vi "Autonomous Independent.vi"() -> ()   [LabVIEW 2015]
doc: "This VI is called when autonomous begins, and will automatically be terminated when autonomous ends. You can carry out timed or sensor driven robot movement independently without needing to return to the caller."
uses:
  AutoStatesTypeDef.ctl
  Auton Defenses Enum.ctl
  <vilib>/Rock Robotics/WPI/Utilities/WPI_GetSetVariantRefNum.vi
  <vilib>/Rock Robotics/Network Tables/NT Read String.vi
  <vilib>/Rock Robotics/Network Tables/NT Write Numeric Array.vi
  <vilib>/Rock Robotics/Network Tables/NT Read Number.vi
  <vilib>/Rock Robotics/Network Tables/NT Write Number.vi
  Robot Values.vi
  Robot Global.vi
  <vilib>/Rock Robotics/Network Tables/NT Read Boolean.vi
  <vilib>/Rock Robotics/WPI/RobotDrive/WPI_RobotDriveArcadeDrive_Standard(NoSaturation).vi
panel:
  in  "PID gains 7":T1={"proportional gain (Kc)"=0.015, "integral time (Ti, min)"=0.0, "derivative time (Td, min)"=0.0}
  in  "PID gains 5":T1={"proportional gain (Kc)"=0.015, "integral time (Ti, min)"=0.0, "derivative time (Td, min)"=0.0}
  in  "PID gains 4":T1={"proportional gain (Kc)"=0.015, "integral time (Ti, min)"=0.0, "derivative time (Td, min)"=0.0}
  in  "PID gains 3":T1={"proportional gain (Kc)"=0.015, "integral time (Ti, min)"=0.0, "derivative time (Td, min)"=0.0}
  in  "Pos 5 Turn":dbl=180.0 format="%#_13g"
  in  "Pos 4 Turn":dbl=180.0 format="%#_13g"
  in  "Pos 3 Turn":dbl=180.0 format="%#_13g"
  in  "Pos 2 Turn":dbl=180.0 format="%#_13g"
  in  "Pos 5 Align":dbl=105.0 format="%#_13g"
  in  "Pos 4 Align":dbl=170.0 format="%#_13g"
  in  "Pos 3 Align":dbl=255.0 format="%#_13g"
  in  "Pos 2 Align":dbl=260.0 format="%#_13g"
  in  "Pos 5 Drive":dbl=-450.0 format="%#_13g"
  in  "Pos 4 Drive":dbl=-50.0 format="%#_13g"
  in  "Pos 3 Drive":dbl=-100.0 format="%#_13g"
  in  "Pos 2 Drive":dbl=-680.0 format="%#_13g"
  in  "PID gains 2":T1={"proportional gain (Kc)"=0.015, "integral time (Ti, min)"=0.0, "derivative time (Td, min)"=0.0}
  in  "Initial State":T2
  in  "Auton":T3={"Position"=enum."First", "Defense"=enum."Low Bar"}
  out "Current Movement, for debugging":T4 {"Y Joystick Value" scale=1.0..-1.0; "X Joystick Value" scale=-1.0..1.0}
  in  "Array of robot movements":T5(array[cluster])=[{"X Joystick Value"=0.39393939393939403, "Y Joystick Value"=0.0, "Delay (sec)"=1.0, "Movement Name"="turn"}, {"X Joystick Value"=-0.3737373737373737, "Y Joystick Value"=0.0, "Delay (sec)"=1.0, "Movement Name"="turn back"}] {"Y Joystick Value" scale=1.0..-1.0; "X Joystick Value" scale=-1.0..1.0}
  # "Be sure to right-click and choose Data Operations>>Make Current Value default if you want to save the array values with the VI"
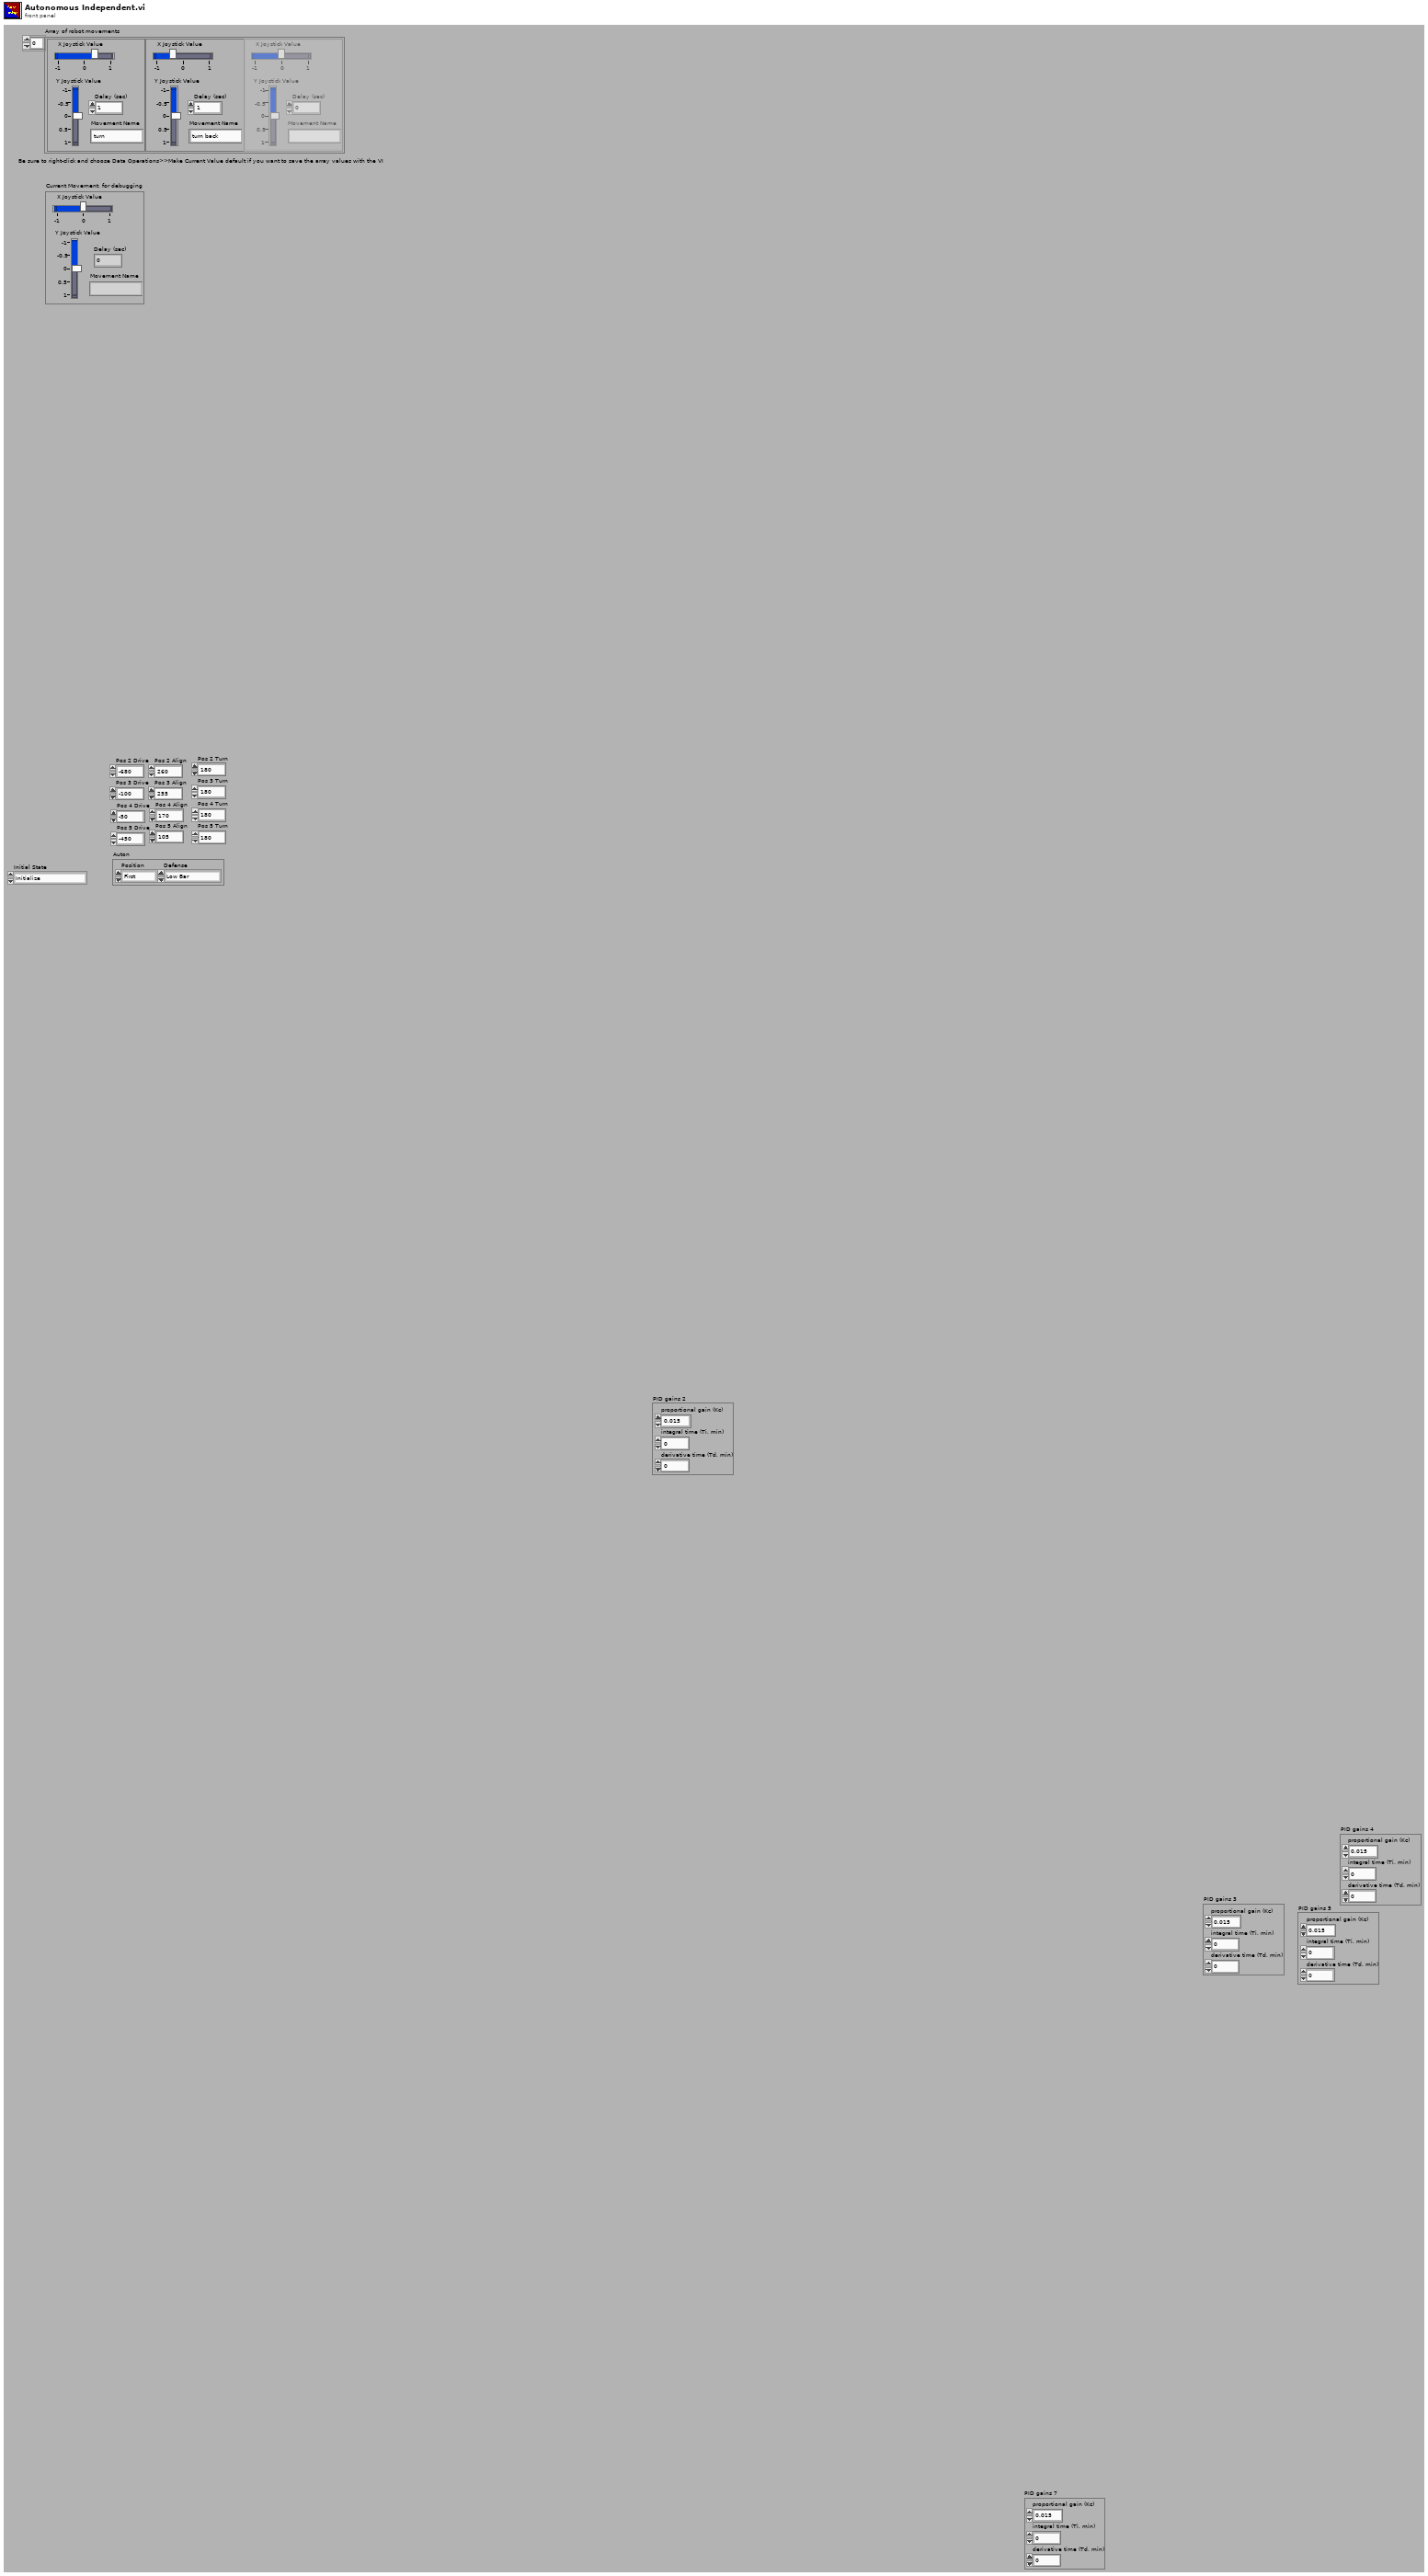
[diagram p1: front panel]
types:
  T1 = cluster{"proportional gain (Kc)":dbl, "integral time (Ti, min)":dbl, "derivative time (Td, min)":dbl}
  T2 = typedef "AutoStatesTypeDef.ctl" = enum16{"Initialize", "Line up to shoot", "Align robot", "Drive to goal", "Lower Arms", "Raise Arms", "Drive to defense", "Cross defense", "Turn towards goal", "Shoot", "Retreat", "Stop"}
  T3 = cluster{"Position":enum16{"First", "Second", "Third", "Fourth", "Fifth"}, "Defense":enum16{"Portcullis", "CDF", "Moat", "Ramparts", "Drawbridge", "Sally Port", "Rock Wall", "Rough Terrain", "Low Bar"}}
  T4 = cluster{"X Joystick Value":dbl, "Y Joystick Value":dbl, "Delay (sec)":dbl, "Movement Name":string}
  T5 = cluster{"X Joystick Value":dbl, "Y Joystick Value":dbl, "Delay (sec)":dbl, "Movement Name":string}[]
  T6 = typedef "WPI_JoystickDevRef.ctl" = cluster{"Device":T7}
  T7 = typedef "WPI_JoystickDeviceEnum.ctl" = enum16{"USB 0", "USB 1", "USB 2", "USB 3", "USB 4", "USB 5"}
  T8 = typedef "Auton Defenses Enum.ctl" = enum16{"Low Bar", "None", "Portcullis", "CDF", "Moat", "Ramparts", "Drawbridge", "Sally Port", "Rock Wall", "Reach", "Spy Bot", "Rough Terrain"}
  T9 = enum16{"First", "Second", "Third", "Fourth", "Fifth"}
  T10 = typedef "Robot Values.ctl" = cluster{"Drive Motors":cluster{"Left Motor Value":dbl, "Right Motor Value":dbl, "Left Motor Encoder":dbl, "Right Motor Encoder":dbl, "High/Low Gear":bool}, "Sensors":cluster{"Gyro Angle":dbl, "Photoeye":bool, "Ultrasonic Range":dbl, "Shooter Speed Encoder":dbl, "Accelerometer Value":dbl, "Flashlight":bool, "Target Distance":dbl, "Target X Value":dbl, "Reset Gyro?":bool}, "Arms":cluster{"Desired Arm Position":dbl, "Left Arm Encoder":dbl, "Right Arm Encoder":dbl, "Left Arm Lower Limit":bool, "Right Arm Lower Limit":bool, "Initialize Arm Position?":bool}, "Acquisition and Scoring":cluster{"Acquiring?":bool, "Current Speed":dbl, "Setpoint Speed":dbl, "Prep Wheels":bool, "Shoot":bool, "Low Eject":bool, "Reverse Shooter Wheel":bool}, "Hanging":cluster{"Pivot Arms":dbl, "PTO":bool, "Left Pivot Encoder":dbl, "Right Pivot Encoder":dbl, "Hanging Pin":bool}}
  T11 = typedef "Robot Drive.ctl" = cluster{"RobotDriveDevRef":T12, "Joysticks":cluster{"JoystickDevRef":T6, "JoystickDevRef 2":T6}, "Sensor":T20, "Pneumatics":T39, "Defenses":cluster{"LeftArm MotorControlDeviceRef":T13, "RightArm MotorControlDeviceRef":T13}, "Hanging":cluster{"Left Erection MotorControlDeviceRef":T13, "Right Erection MotorControlDeviceRef":T13}, "Aquisition + Scoring":T43, "DigitalOutputDevRef":T47, "DigitalInputDevRef":T24}
  T12 = typedef "WPI_RobotDriveDevRef.ctl" = cluster{"DevStatus":errorcluster, "Motors[]":T13[], "Square Inputs":bool, "Max Output":dbl}
  T13 = typedef "WPI_MotorControlDeviceRef.ctl" = cluster{"DeviceStatus":errorcluster, "Type":T14, "PWM":cluster{"PWM Channel":T15, "DeadBand":T16}, "CAN":cluster{"Device Number":u8, "Control Mode":T17, "Semaphore":T18, "Max Vout":dbl, "TalonSRX Control Mode":T19}, "Invert":bool}
  T14 = typedef "WPI_MotorControlType.ctl" = enum16{"PWM", "CAN", "CANTalonSRX"}
  T15 = typedef "FPGA_DIOPWMChannel.ctl" = enum8{"PWM 0", "PWM 1", "PWM 2", "PWM 3", "PWM 4", "PWM 5", "PWM 6", "PWM 7", "PWM 8", "PWM 9", "PWM MXP 0", "PWM MXP 1", "PWM MXP 2", "PWM MXP 3", "PWM MXP 4", "PWM MXP 5", "PWM MXP 6", "PWM MXP 7", "PWM MXP 8", "PWM MXP 9", "Invalid"}
  T16 = typedef "WPI_PWMDeadband.ctl" = cluster{"Name":string, "maxPositivePwm":i32, "minPositivePwm":i32, "centerPwm":i32, "maxNegativePwm":i32, "minNegativePwm":i32, "angularRange":u16}
  T17 = typedef "WPI_CANJaguar_ControlMode.ctl" = enum8{"Percent VBus", "Current", "Speed", "Position", "Voltage"}
  T18 = typedef "Semaphore RefNum" = refnum<k1>
  T19 = typedef "WPI_CANTalonSRX_APIControlMode.ctl" = enum8{"Percent VBus", "Speed", "Position", "Slave", "Unchanged / Invalid", "Voltage Compensation", "Current", "Motion Profile"}
  T20 = typedef "Sensors.ctl" = cluster{"GyroDevRef":T21, "Left Arm Limit DigitalInputDevRef":T24, "Right Arm Limit DigitalInputDevRef":T24, "Left Arm EncoderDevRef":T26, "Right Arm EncoderDevRef":T26, "Left Drive EncoderDevRef":T26, "Right Drive EncoderDevRef":T26, "BoB Photoeye DigitalInputDevRef":T24, "Range SonarMB1010AnalogDevRef":T30, "Shooter CounterDevRef":T32, "AccelerometerDevRef":T33, "Left Hanging Erecter EncoderDevRef":T26, "Right Hanging Erecter EncoderDevRef":T26, "TestDigitalInputDevRef":T24}
  T21 = typedef "WPI_GyroDevRef.ctl" = cluster{"DevStatus":errorcluster, "Analog Channel":T22, "Offset":dbl, "Gain (VoltsPerDegree/Second)":dbl, "Gyro Type":enum16{"Analog", "XRS450"}, "Handle":i32, "SPI Bus":T23, "Device Found":bool, "Sample Rate":dbl, "Calibrate On Open":bool}
  T22 = typedef "FPGA_AIChannel.ctl" = enum8{"AI 0", "AI 1", "AI 2", "AI 3", "AI MXP 0", "AI MXP 1", "AI MXP 2", "AI MXP 3", "Invalid"}
  T23 = typedef "spi_bus.ctl" = enum16{"SPI On-Board, CS0", "SPI On-Board, CS1", "SPI On-Board, CS2", "SPI On-Board, CS3", "SPI MXP", "Invalid"}
  T24 = typedef "WPI_DigitalInputDevRef.ctl" = cluster{"DevStatus":errorcluster, "DIO Channel":T25}
  T25 = typedef "FPGA_DIOChannel.ctl" = enum8{"DIO 0", "DIO 1", "DIO 2", "DIO 3", "DIO 4", "DIO 5", "DIO 6", "DIO 7", "DIO 8", "DIO 9", "DIO MXP 0", "DIO MXP 1", "DIO MXP 2", "DIO MXP 3", "DIO MXP 4", "DIO MXP 5", "DIO MXP 6", "DIO MXP 7", "DIO MXP 8", "DIO MXP 9", "DIO MXP 10", "DIO MXP 11", "DIO MXP 12", "DIO MXP 13", "DIO MXP 14", "DIO MXP 15", "Invalid"}
  T26 = typedef "WPI_EncoderDevRef.ctl" = cluster{"DevStatus":errorcluster, "EncoderIndex":T27, "CounterIndex":T28, "DistancePerCount":dbl, "Decoding Type":T29}
  T27 = typedef "FPGA_EncoderIdx.ctl" = enum8{"Enc 0", "Enc 1", "Enc 2", "Enc 3", "Enc 4", "Enc 5", "Enc 6", "Enc 7", "Invalid"}
  T28 = typedef "FPGA_CounterCtrSystemIndex.ctl" = enum8{"Ctr 0", "Ctr 1", "Ctr 2", "Ctr 3", "Ctr 4", "Ctr 5", "Ctr 6", "Ctr 7", "Invalid"}
  T29 = typedef "WPI_EncoderType.ctl" = enum16{"1x", "2x", "4x"}
  T30 = typedef "WPI_SonarMB1010AnalogDeviceRef.ctl" = cluster{"AIDeviceRef":T31, "Scaling factor (V/in)":dbl, "Average Bits":u8}
  T31 = typedef "WPI_AnalogChannelDevRef.ctl" = cluster{"DevStatus":errorcluster, "Analog Channel":T22}
  T32 = typedef "WPI_CounterDevRef.ctl" = cluster{"DevStatus":errorcluster, "CntIndex":T28}
  T33 = typedef "WPI_AccelerometerDevRef.ctl" = cluster{"DevStatus":errorcluster, "Scaling":T34, "Analog Channels":T35, "I2C Bus":T36, "SPI Bus":T23, "Accel Range":T37, "ADXL Axes":T38, "Handle":i32, "Device Address":u8, "Accel Type":enum16{"Analog", "ADXL345 I2C", "ADXL345 SPI", "Internal", "ADXL362 SPI"}}
  T34 = typedef "WPI_AccelerometerScaling.ctl" = cluster{"Gain (VoltsPerG)":dbl, "Center Voltage":dbl}
  T35 = typedef "WPI_AccelerometerAnalogChannels.ctl" = cluster{"X-Axis":T22, "Y-Axis":T22, "Z-Axis":T22}
  T36 = typedef "i2c_bus.ctl" = enum16{"I2C On-Board", "I2C MXP", "Invalid"}
  T37 = typedef "ADXL345 Range.ctl" = u8
  T38 = typedef "WPI_AccelerometerADXL345 Axes.ctl" = cluster{"X-Axis":bool, "Y-Axis":bool, "Z-Axis":bool}
  T39 = typedef "Pnematics.ctl" = cluster{"CompressorDevRef":T40, "High and Low Gear DoubleSolenoidDevRef":T41, "PTO SolenoidDevRef":T41, "Hang Pin SolenoidDevRef":T41}
  T40 = typedef "WPI_CompressorDevRef.ctl" = cluster{"DevStatus":errorcluster, "Pneumatics Control Module":u8}
  T41 = typedef "WPI_SolenoidDevRef.ctl" = cluster{"DevStatus":errorcluster, "Pneumatics Control Module":u8, "Forward Solenoid Channel":T42, "Reverse Solenoid Channel":T42}
  T42 = typedef "WPI_SolenoidChannel.ctl" = enum8{"Solenoid 0", "Solenoid 1", "Solenoid 2", "Solenoid 3", "Solenoid 4", "Solenoid 5", "Solenoid 6", "Solenoid 7", "Invalid"}
  T43 = typedef "Acquisition & Scoring.ctl" = cluster{"Outer Roller MotorControlDeviceRef":T13, "Inner Roller MotorControlDeviceRef":T13, "Scoring Top MotorControlDeviceRef":T13, "Scoring Bottom MotorControlDeviceRef":T13, "Flashlight RelayDevRef":T44}
  T44 = typedef "WPI_RelayDevRef.ctl" = cluster{"DevStatus":errorcluster, "Relay Channel":T45, "Relay Direction":T46}
  T45 = typedef "FPGA_DIORelayChannel.ctl" = enum8{"Relay 0", "Relay 1", "Relay 2", "Relay 3", "Invalid"}
  T46 = typedef "WPI_RelayDirection.ctl" = enum16{"Both directions", "Forward only", "Reverse only"}
  T47 = typedef "WPI_DigitalOutputDevRef.ctl" = cluster{"DIO Channel":T25, "DevStatus":errorcluster}
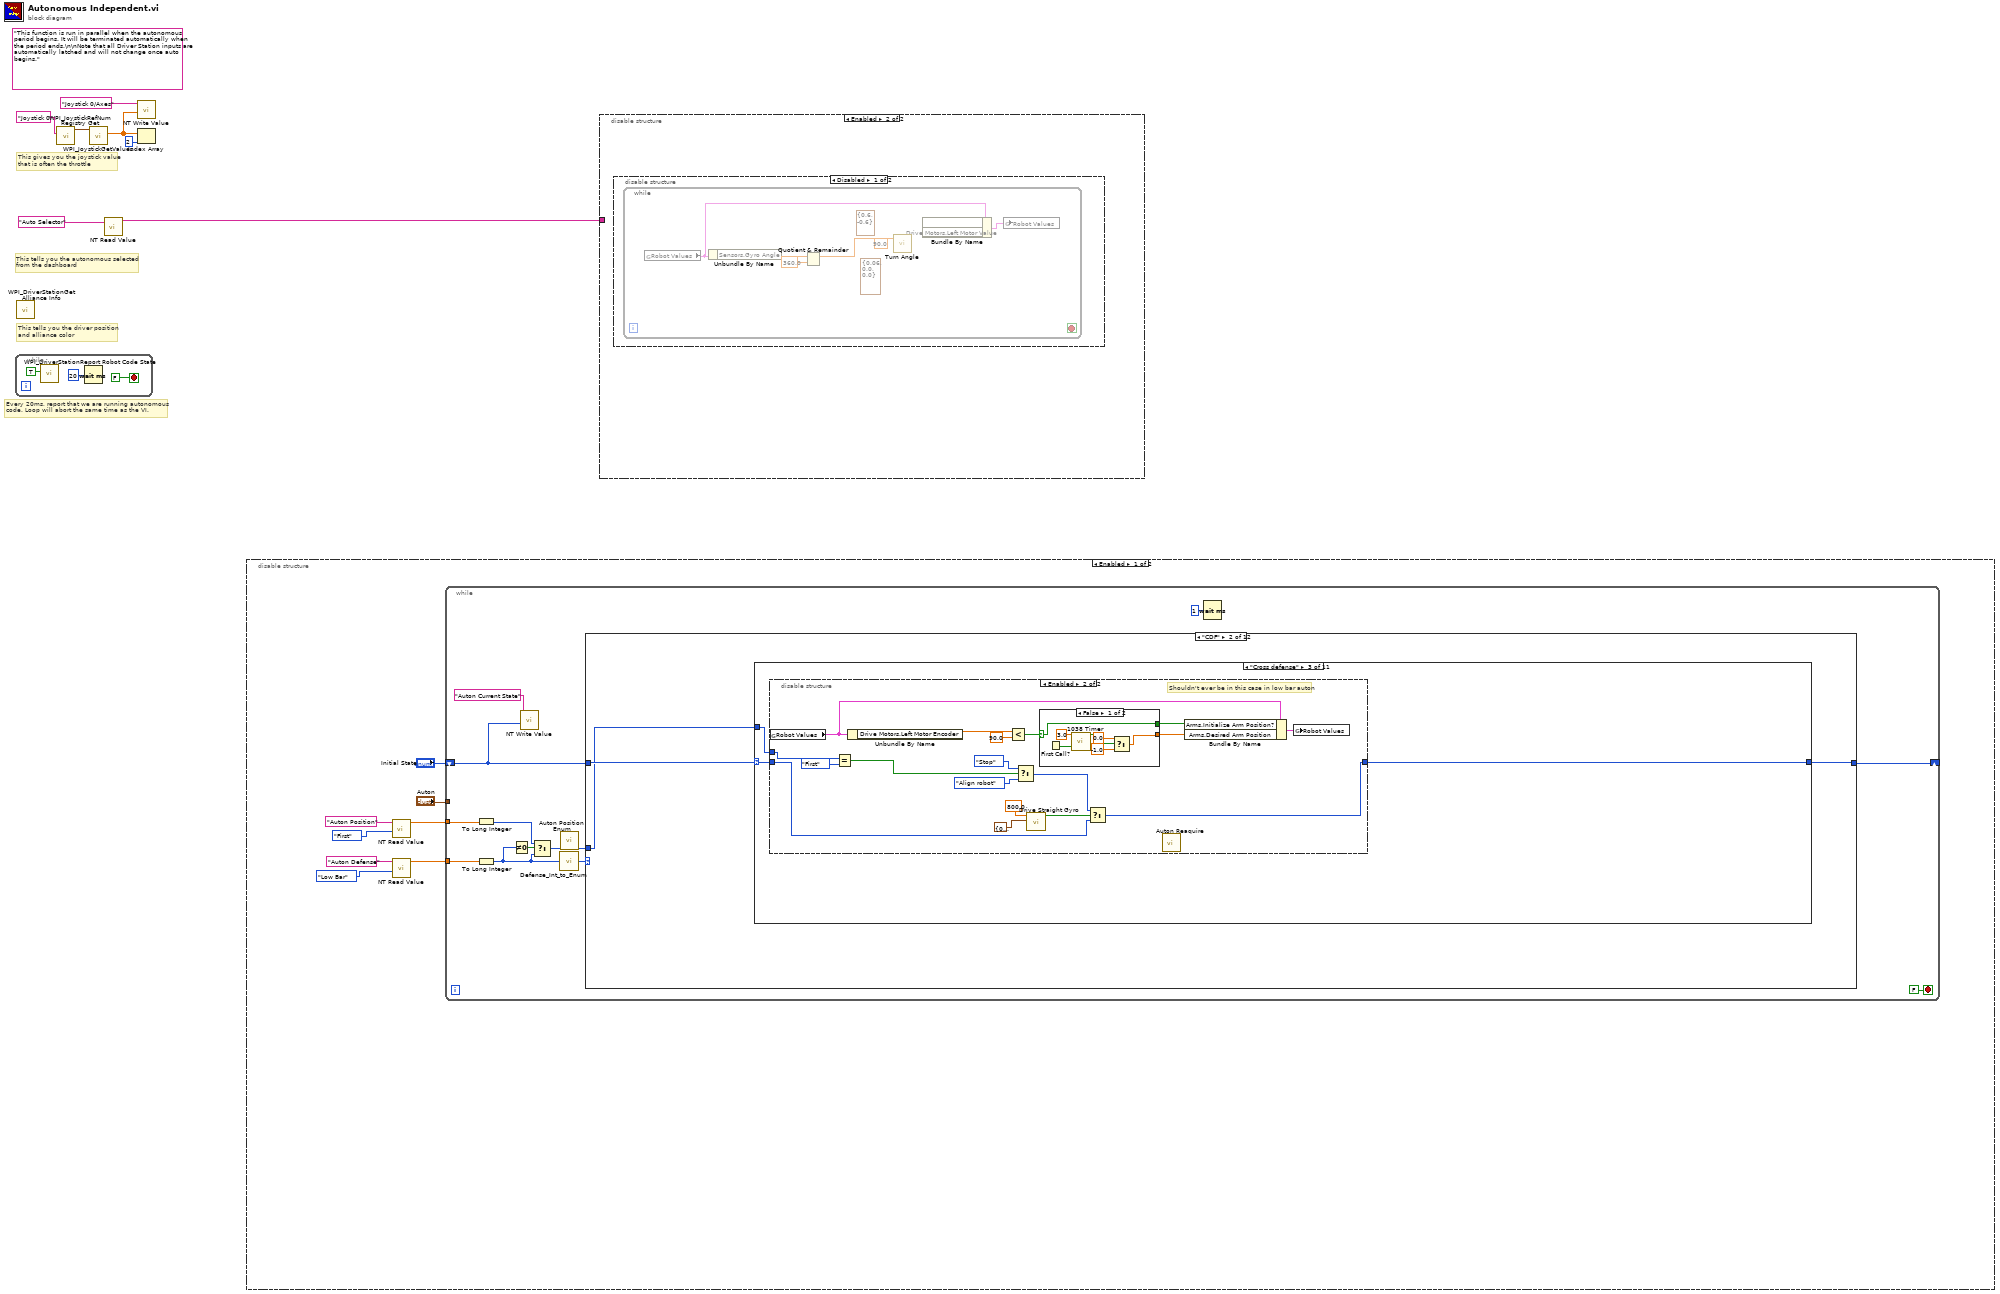
[diagram p0: block diagram]
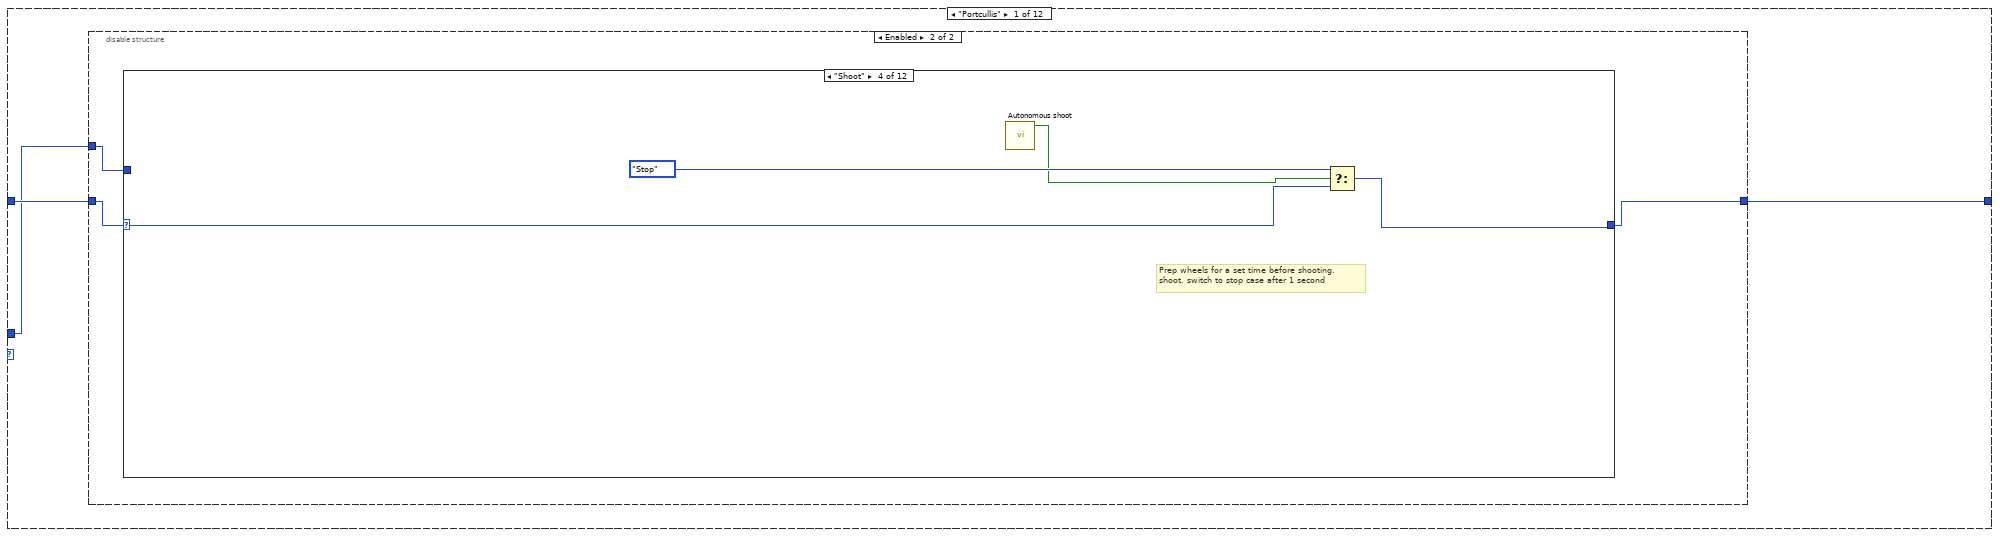
[diagram p2: hidden frame]
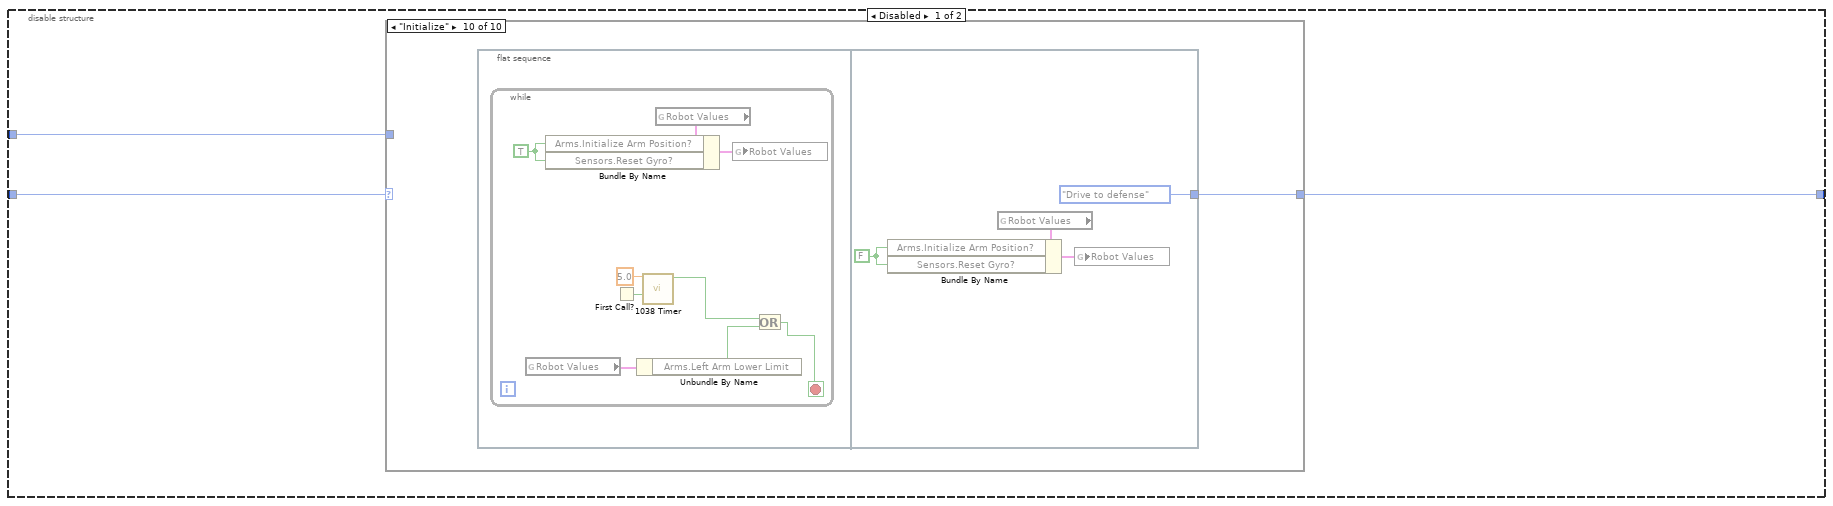
[diagram p3: hidden frame]
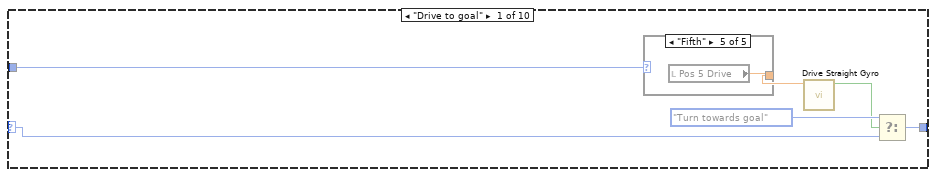
[diagram p4: hidden frame]
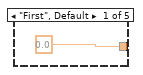
[diagram p5: hidden frame]
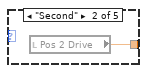
[diagram p6: hidden frame]
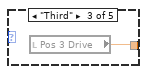
[diagram p7: hidden frame]
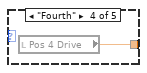
[diagram p8: hidden frame]
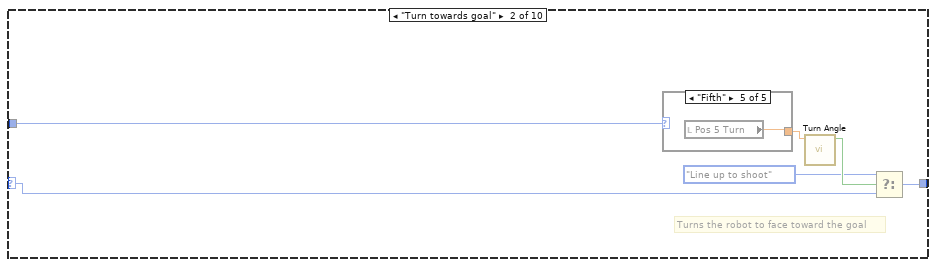
[diagram p9: hidden frame]
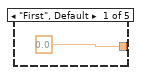
[diagram p10: hidden frame]
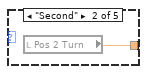
[diagram p11: hidden frame]
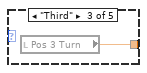
[diagram p12: hidden frame]
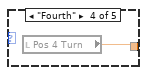
[diagram p13: hidden frame]
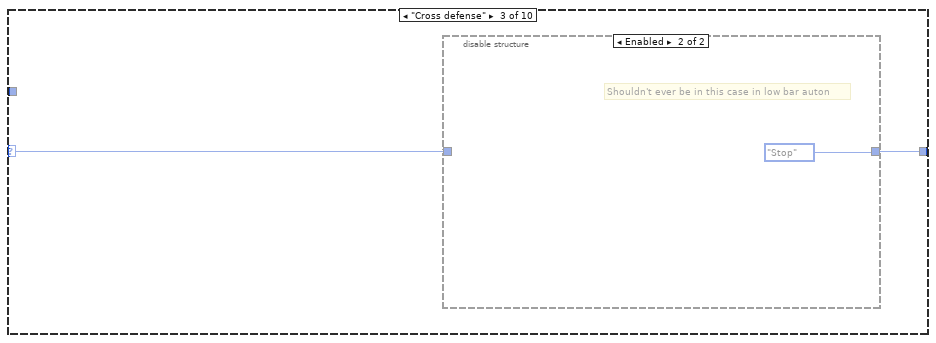
[diagram p14: hidden frame]
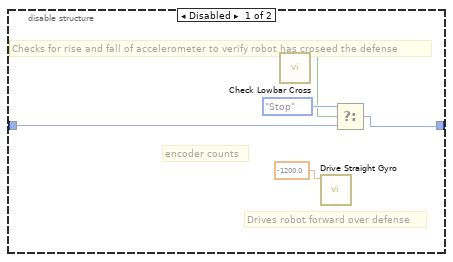
[diagram p15: hidden frame]
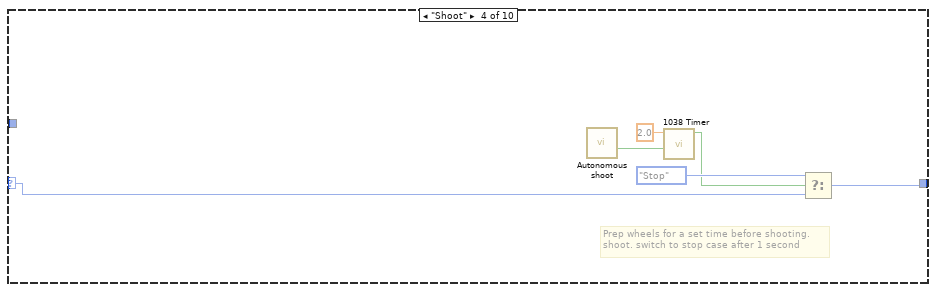
[diagram p16: hidden frame]
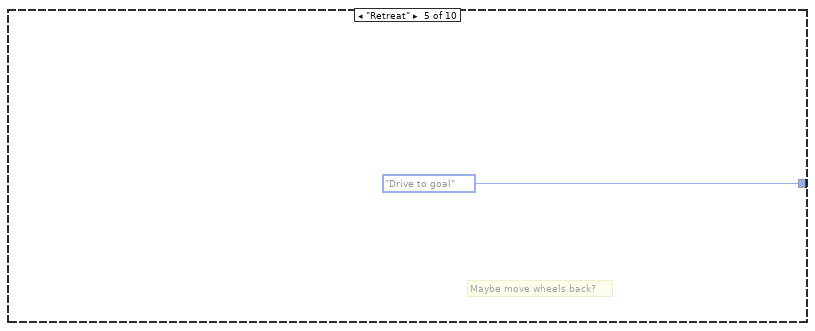
[diagram p17: hidden frame]
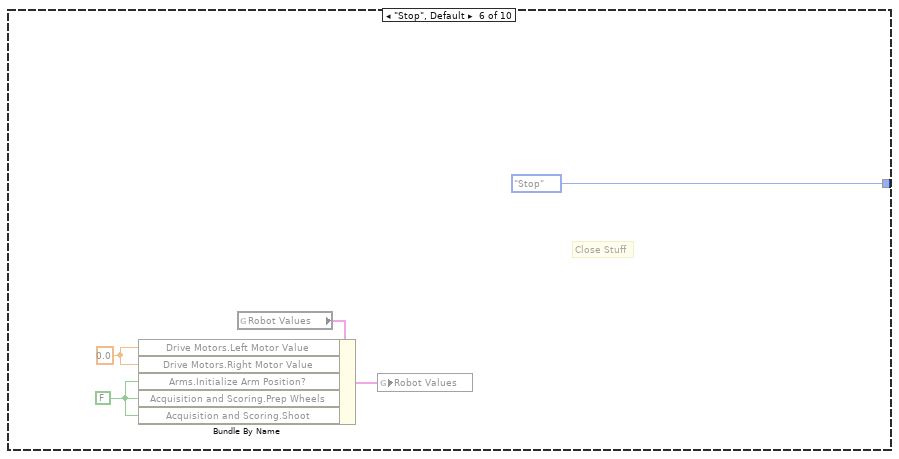
[diagram p18: hidden frame]
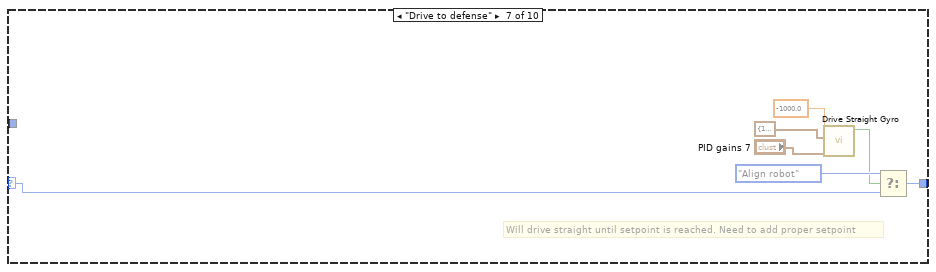
[diagram p19: hidden frame]
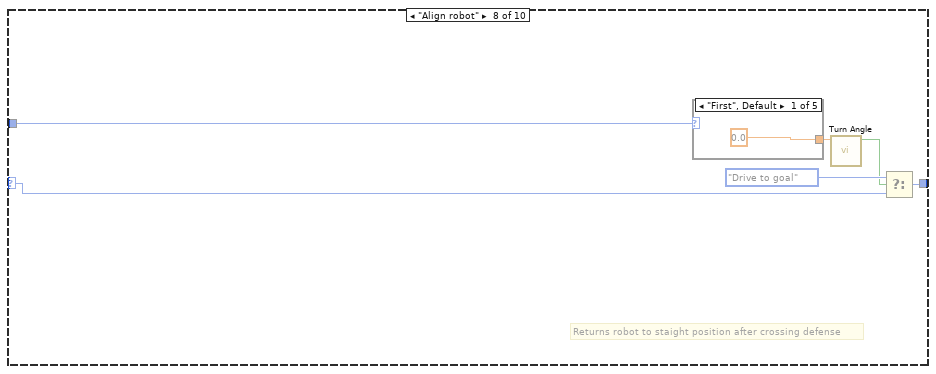
[diagram p20: hidden frame]
diagram:
  (unwired) "This function is run in parallel when the autonomous period begins. It will be terminated automatically when the period ends.\n\nNote that all Driver Station inputs are automatically latched and will not change once auto begins."
  # "This tells you the autonomous selected\nfrom the dashboard"
  # "Every 20ms, report that we are running autonomous\ncode. Loop will abort the same time as the VI."
  # "This gives you the joystick value\nthat is often the throttle"
  # "This tells you the driver position\nand alliance color"
  n1 = while {
    stop <- FALSE stop-if-true
    n2 = call <vilib>:"WPI_DriverStationReport Robot Code State.vi"("Autonomous"=TRUE) -> ()  [unwired: 10 in, 1 out]
    n3 = Wait (ms)(milliseconds to wait=u32 20) -> ()  [unwired: 1 out]
  }
  n4 = call <vilib>:"WPI_DriverStationGet Alliance Info.vi"() -> ()  [unwired: 12 out]
  n5 = call <vilib>:"WPI_JoystickRefNum Registry Get.vi"("refnum name"="Joystick 0") -> ("JoystickDevRef"=w6:T6)  [unwired: 1 in, 9 out]
  n6 = call <vilib>:"WPI_JoystickGetValues.vi"("JoystickDevRef"=w6) -> ("Axes"=w2:dbl[])  [unwired: 6 in, 4 out]
  n7 = call-poly <vilib>:"NT Read Value.vi"("Name"="Auto Selector") -> ("String"=w3:string)  [unwired: 9 in, 1 out]
  n8 = call-poly <vilib>:"NT Write Value.vi"("Numeric Array"=w2, "Name"="Joystick 0/Axes") -> ()  [unwired: 9 in, 1 out]
  n9 = Index Array(array=w2, index=2) -> ()  [unwired: 1 out]
  n10 = disable-structure shown="Enabled" {
    frame Enabled {
      n11 = call-poly <vilib>:"NT Read Value.vi"("Default Value"=T9."First" ("Position"), "Name"="Auton Position") -> ("Numeric"=w13:dbl)  [unwired: 8 in, 1 out]
      n12 = call-poly <vilib>:"NT Read Value.vi"("Default Value"=Auton_Defenses_Enum."Low Bar" ("Defense"), "Name"="Auton Defense") -> ("Numeric"=w14:dbl)  [unwired: 8 in, 1 out]
      n13 = while {
        tunnel: "Auton" -> [_]
        tunnel: w14 -> [w30]
        tunnel: w13 -> [w31]
        shift-right: [w28] -> _
        shift-left: "Initial State" -> [w20]
        stop <- FALSE stop-if-true
        n14 = To Long Integer(number=w31) -> (32bit integer=w24:i32)
        n15 = To Long Integer(number=w30) -> (32bit integer=w25:i32)
        n16 = Not Equal To 0?(x=w25) -> (x != 0?=w26:bool)
        n17 = call-poly <vilib>:"NT Write Value.vi"("Numeric"=w20, "Name"="Auton Current State") -> ()  [unwired: 9 in, 1 out]
        n18 = Select(t=w24, s=w26, f=w25) -> (s? t:f=w23:i32)
        n19 = call "Defense_Int_to_Enum.vi"("Defense"=w25) -> ("Defense"=w27:T8)
        n20 = call "Auton Position Enum.vi"("Position"=w23) -> ("Position"=w22:T9)  [unwired: 10 in]
        n21 = case shown="\"CDF\"" w27 {
          tunnel: [w32 w282 w474 w558 _ _ w642 w767 w916 _ w1032 _] -> w28
          tunnel: w22 -> [w33 w283 w475 w559 _ _ w643 w768 _ _ _ _]
          tunnel: w20 -> [w34 w284 w476 w560 _ _ w644 w766 w915 _ w1033 _]
          frame "Portcullis" {
            n22 = disable-structure shown="Enabled" {
              disable-tunnel: w34 -> [w37 w121]
              disable-tunnel: w33 -> [w36 w119]
              disable-tunnel: [w35 w120] -> w32
              frame Disabled {
                n23 = case shown="\"Initialize\"" w37 {
                  selector: w37 -> [w41 w52 w60 w70 _ _ w82 w92 w101 _]
                  tunnel: [w43 w54 w61 w69 AutoStatesTypeDef."Drive to goal" ("Defense") AutoStatesTypeDef."Stop" ("Defense") w85 w91 w104 w105] -> w35
                  tunnel: w36 -> [w39 w50 _ _ _ _ _ w87 _ _]
                  frame "Drive to goal" {
                    n24 = case shown="\"Fifth\"" w39 {
                      tunnel: [0.0 ("setpoint") w45 w46 w47 w48] -> w38
                      frame "First", Default {
                      }
                      frame "Second" {
                        n25 = local read "Pos 2 Drive"() -> (w45:dbl)
                      }
                      frame "Third" {
                        n26 = local read "Pos 3 Drive"() -> (w46:dbl)
                      }
                      frame "Fourth" {
                        n27 = local read "Pos 4 Drive"() -> (w47:dbl)
                      }
                      frame "Fifth" {
                        n28 = local read "Pos 5 Drive"() -> (w48:dbl)
                      }
                    }
                    n29 = call "Drive Straight Gyro.vi"("Distance to travel"=w38) -> ("In Range?"=w40:bool)  [unwired: 10 in]
                    n30 = Select(t=AutoStatesTypeDef."Turn towards goal", s=w40, f=w41) -> (s? t:f=w43:T2)
                  }
                  frame "Turn towards goal" {
                    # "Turns the robot to face toward the goal"
                    n31 = case shown="\"Fifth\"" w50 {
                      tunnel: [0.0 ("setpoint") w56 w57 w58 w59] -> w49
                      frame "First", Default {
                      }
                      frame "Second" {
                        n32 = local read "Pos 2 Turn"() -> (w56:dbl)
                      }
                      frame "Third" {
                        n33 = local read "Pos 3 Turn"() -> (w57:dbl)
                      }
                      frame "Fourth" {
                        n34 = local read "Pos 4 Turn"() -> (w58:dbl)
                      }
                      frame "Fifth" {
                        n35 = local read "Pos 5 Turn"() -> (w59:dbl)
                      }
                    }
                    n36 = call "Turn Angle.vi"("setpoint"=w49) -> ("In Range?"=w53:bool)  [unwired: 10 in]
                    n37 = Select(t=AutoStatesTypeDef."Line up to shoot" ("Defense"), s=w53, f=w52) -> (s? t:f=w54:T2)
                  }
                  frame "Cross defense" {
                    n38 = disable-structure shown="Enabled" {
                      disable-tunnel: [w66 AutoStatesTypeDef."Stop" ("Defense")] -> w61
                      disable-tunnel: w60 -> [w64 _]
                      frame Disabled {
                        # "Checks for rise and fall of accelerometer to verify robot has croseed the defense"
                        # "Drives robot forward over defense"
                        # "encoder counts"
                        n39 = call "Check Lowbar Cross.vi"() -> ("Cross"=w63:bool)  [unwired: 11 in]
                        n40 = call "Drive Straight Gyro.vi"("Distance to travel"=-1200.0) -> ()  [unwired: 10 in, 1 out]
                        n41 = Select(t=AutoStatesTypeDef."Stop" ("Defense"), s=w63, f=w64) -> (s? t:f=w66:T2)
                      }
                      frame Enabled {
                        # "Shouldn't ever be in this case in low bar auton"
                      }
                    }
                  }
                  frame "Shoot" {
                    # "Prep wheels for a set time before shooting.\nshoot. switch to stop case after 1 second"
                    n42 = call "Autonomous shoot.vi"() -> ("Shot?"=w72:bool)  [unwired: 11 in]
                    n43 = call "1038 Timer.vi"("Reset?"=w72, "Time Target"=2.0) -> ("Done?"=w68:bool)  [unwired: 9 in]
                    n44 = Select(t=AutoStatesTypeDef."Stop" ("Defense"), s=w68, f=w70) -> (s? t:f=w69:T2)
                  }
                  frame "Retreat" {
                    # "Maybe move wheels back?"
                  }
                  frame "Stop", Default {
                    w75 = FALSE ("Arms.Initialize Arm Position?")
                    w76 = 0.0
                    # "Close Stuff"
                    n45 = global read "Robot Values.vi" "Robot Values"() -> (w78:T10)
                    n46 = Bundle By Name(cluster=w78, "Drive Motors.Left Motor Value"=w76, "Drive Motors.Right Motor Value"=w76, "Arms.Initialize Arm Position?"=w75, "Acquisition and Scoring.Prep Wheels"=w75, "Acquisition and Scoring.Shoot"=w75) -> (w77:T10)
                    n47 = global write "Robot Values.vi" "Robot Values"(w77) -> ()
                  }
                  frame "Drive to defense" {
                    # "Will drive straight until setpoint is reached. Need to add proper setpoint"
                    n48 = call "Drive Straight Gyro.vi"("PID gains"="PID gains 7", "output range"=cluster{"output high":dbl, "output low":dbl} {"output high"=1.0, "output low"=-1.0}, "Distance to travel"=-1000.0) -> ("In Range?"=w83:bool)  [unwired: 8 in]
                    n49 = Select(t=AutoStatesTypeDef."Align robot" ("Defense"), s=w83, f=w82) -> (s? t:f=w85:T2)
                  }
                  frame "Align robot" {
                    # "Returns robot to staight position after crossing defense"
                    n50 = case shown="\"First\", Default" w87 {
                      tunnel: [0.0 ("setpoint") w94 w95 w96 w97] -> w89
                      frame "First", Default {
                      }
                      frame "Second" {
                        n51 = local read "Pos 2 Align"() -> (w94:dbl)
                      }
                      frame "Third" {
                        n52 = local read "Pos 3 Align"() -> (w95:dbl)
                      }
                      frame "Fourth" {
                        n53 = local read "Pos 4 Align"() -> (w96:dbl)
                      }
                      frame "Fifth" {
                        n54 = local read "Pos 5 Align"() -> (w97:dbl)
                      }
                    }
                    n55 = call "Turn Angle.vi"("setpoint"=w89) -> ("In Range?"=w88:bool)  [unwired: 10 in]
                    n56 = Select(t=AutoStatesTypeDef."Drive to goal" ("Defense"), s=w88, f=w92) -> (s? t:f=w91:T2)
                  }
                  frame "Line up to shoot" {
                    n57 = call "Align to Shoot.vi"() -> ("Stop?"=w98:bool, "Aligned?"=w102:bool)  [unwired: 10 in]
                    n58 = Select(t=AutoStatesTypeDef."Stop" ("Defense"), s=w98, f=w101) -> (s? t:f=w100:T2)
                    n59 = Select(t=AutoStatesTypeDef."Shoot" ("Defense"), s=w102, f=w100) -> (s? t:f=w104:T2)
                  }
                  frame "Initialize" {
                    n60 = flat-sequence {
                      tunnel: [AutoStatesTypeDef."Drive to defense" ("t")] -> w105
                      frame #0 {
                        n61 = while {
                          stop <- w109 stop-if-true
                          w111 = TRUE ("Arms.Initialize Arm Position?")
                          n62 = global read "Robot Values.vi" "Robot Values"() -> (w112:T10)
                          n63 = First Call?() -> (First Call?: T/F=w108:bool)
                          n64 = Unbundle By Name(w112) -> ("Arms.Left Arm Lower Limit"=w110:bool)
                          n65 = call "1038 Timer.vi"("Reset?"=w108, "Time Target"=5.0) -> ("Done?"=w106:bool)  [unwired: 9 in]
                          n66 = global read "Robot Values.vi" "Robot Values"() -> (w114:T10)
                          n67 = Bundle By Name(cluster=w114, "Arms.Initialize Arm Position?"=w111, "Sensors.Reset Gyro?"=w111) -> (w113:T10)
                          n68 = global write "Robot Values.vi" "Robot Values"(w113) -> ()
                          n69 = Or(x=w106, y=w110) -> (x .or. y?=w109:bool)
                        }
                      }
                      frame #1 {
                        w118 = FALSE ("Arms.Initialize Arm Position?")
                        n70 = global read "Robot Values.vi" "Robot Values"() -> (w116:T10)
                        n71 = Bundle By Name(cluster=w116, "Arms.Initialize Arm Position?"=w118, "Sensors.Reset Gyro?"=w118) -> (w117:T10)
                        n72 = global write "Robot Values.vi" "Robot Values"(w117) -> ()
                      }
                    }
                  }
                }
              }
              frame Enabled {
                n73 = case shown="\"Shoot\"" w121 {
                  selector: w121 -> [w125 w136 w145 w172 _ _ w182 w193 w219 _ _ _]
                  tunnel: [w127 w138 w146 w171 AutoStatesTypeDef."Drive to goal" ("Defense") AutoStatesTypeDef."Stop" ("Defense") w185 w192 w222 w223 w238 w260] -> w120
                  tunnel: w119 -> [w123 w134 w144 _ _ _ _ w189 _ _ _ _]
                  frame "Drive to goal" {
                    n74 = case shown="\"Fifth\"" w123 {
                      tunnel: [0.0 ("setpoint") w129 w130 w131 w132] -> w122
                      frame "First", Default {
                      }
                      frame "Second" {
                        n75 = local read "Pos 2 Drive"() -> (w129:dbl)
                      }
                      frame "Third" {
                        n76 = local read "Pos 3 Drive"() -> (w130:dbl)
                      }
                      frame "Fourth" {
                        n77 = local read "Pos 4 Drive"() -> (w131:dbl)
                      }
                      frame "Fifth" {
                        n78 = local read "Pos 5 Drive"() -> (w132:dbl)
                      }
                    }
                    n79 = call "Drive Straight Gyro.vi"("Distance to travel"=w122) -> ("In Range?"=w124:bool)  [unwired: 10 in]
                    n80 = Select(t=AutoStatesTypeDef."Turn towards goal", s=w124, f=w125) -> (s? t:f=w127:T2)
                  }
                  frame "Turn towards goal" {
                    # "Turns the robot to face toward the goal"
                    n81 = case shown="\"Fifth\"" w134 {
                      tunnel: [0.0 ("setpoint") w140 w141 w142 w143] -> w133
                      frame "First", Default {
                      }
                      frame "Second" {
                        n82 = local read "Pos 2 Turn"() -> (w140:dbl)
                      }
                      frame "Third" {
                        n83 = local read "Pos 3 Turn"() -> (w141:dbl)
                      }
                      frame "Fourth" {
                        n84 = local read "Pos 4 Turn"() -> (w142:dbl)
                      }
                      frame "Fifth" {
                        n85 = local read "Pos 5 Turn"() -> (w143:dbl)
                      }
                    }
                    n86 = call "Turn Angle.vi"("setpoint"=w133) -> ("In Range?"=w137:bool)  [unwired: 10 in]
                    n87 = Select(t=AutoStatesTypeDef."Line up to shoot" ("Defense"), s=w137, f=w136) -> (s? t:f=w138:T2)
                  }
                  frame "Cross defense" {
                    n88 = disable-structure shown="Enabled" {
                      disable-tunnel: [w151 w165] -> w146
                      disable-tunnel: w145 -> [w149 w166]
                      disable-tunnel: w144 -> [_ w157]
                      frame Disabled {
                        # "Checks for rise and fall of accelerometer to verify robot has croseed the defense"
                        # "Drives robot forward over defense"
                        # "encoder counts"
                        n89 = call "Check Lowbar Cross.vi"() -> ("Cross"=w148:bool)  [unwired: 11 in]
                        n90 = call "Drive Straight Gyro.vi"("Distance to travel"=-1200.0) -> ()  [unwired: 10 in, 1 out]
                        n91 = Select(t=AutoStatesTypeDef."Stop" ("Defense"), s=w148, f=w149) -> (s? t:f=w151:T2)
                      }
                      frame Enabled {
                        n92 = Equal?(x=w157, y=T9."Third") -> (x = y?=w155:bool)
                        n93 = Select(t=AutoStatesTypeDef."Align robot", s=w155, f=AutoStatesTypeDef."Stop" ("t")) -> (s? t:f=w152:T2)
                        n94 = call "Drive Straight Gyro.vi"("output range"=cluster{"output high":dbl, "output low":dbl} {"output high"=0.6, "output low"=-0.6}, "Distance to travel"=600.0) -> ("In Range?"=w167:bool)  [unwired: 9 in]
                        n95 = First Call?() -> (First Call?: T/F=w163:bool)
                        n96 = call "1038 Timer.vi"("Reset?"=w163, "Time Target"=3.0) -> ("Done?"=w161:bool)  [unwired: 9 in]
                        n97 = Select(t=w152, s=w167, f=w166) -> (s? t:f=w165:T2)
                        n98 = Select(t=0.0, s=w161, f=-1.0) -> (s? t:f=w164:dbl)
                        n99 = call "Auton Reaquire.vi"() -> ()  [unwired: 12 in]
                        n100 = global read "Robot Values.vi" "Robot Values"() -> (w169:T10)
                        n101 = Bundle By Name(cluster=w169, "Arms.Desired Arm Position"=w164) -> (w170:T10)
                        n102 = global write "Robot Values.vi" "Robot Values"(w170) -> ()
                      }
                    }
                  }
                  frame "Shoot" {
                    # "Prep wheels for a set time before shooting.\nshoot. switch to stop case after 1 second"
                    n103 = call "Autonomous shoot.vi"() -> ("Shot?"=w173:bool)  [unwired: 11 in]
                    n104 = Select(t=AutoStatesTypeDef."Stop" ("Defense"), s=w173, f=w172) -> (s? t:f=w171:T2)
                  }
                  frame "Retreat" {
                    # "Maybe move wheels back?"
                  }
                  frame "Stop", Default {
                    w176 = FALSE ("Arms.Initialize Arm Position?")
                    w177 = 0.0
                    # "Close Stuff"
                    n105 = global read "Robot Values.vi" "Robot Values"() -> (w179:T10)
                    n106 = Bundle By Name(cluster=w179, "Drive Motors.Left Motor Value"=w177, "Drive Motors.Right Motor Value"=w177, "Arms.Initialize Arm Position?"=w176, "Acquisition and Scoring.Prep Wheels"=w176, "Acquisition and Scoring.Shoot"=w176) -> (w178:T10)
                    n107 = global write "Robot Values.vi" "Robot Values"(w178) -> ()
                  }
                  frame "Drive to defense" {
                    # "Will drive straight until setpoint is reached. Need to add proper setpoint"
                    n108 = call "Drive Straight Gyro.vi"("output range"=cluster{"output high":dbl, "output low":dbl} {"output high"=0.6, "output low"=-0.6}, "Distance to travel"=180.0) -> ("In Range?"=w183:bool)  [unwired: 9 in]
                    n109 = Select(t=AutoStatesTypeDef."Lower Arms" ("Defense"), s=w183, f=w182) -> (s? t:f=w185:T2)
                  }
                  frame "Align robot" {
                    # "Turns the robot around to face toward the goal"
                    n110 = case shown="\"Third\"" w189 {
                      tunnel: [0.0 ("setpoint") w210 w211 w214 w215] -> w190
                      frame "First", Default {
                      }
                      frame "Second" {
                        n111 = local read "Pos 2 Align"() -> (w210:dbl)
                      }
                      frame "Third" {
                        n112 = disable-structure shown="Enabled" {
                          disable-tunnel: [w212 180.0 ("Pos 3 Align")] -> w211
                          frame Enabled {
                            n113 = local read "Pos 3 Align"() -> (w212:dbl)
                          }
                          frame Disabled {
                          }
                        }
                      }
                      frame "Fourth" {
                        n114 = local read "Pos 4 Align"() -> (w214:dbl)
                      }
                      frame "Fifth" {
                        n115 = local read "Pos 5 Align"() -> (w215:dbl)
                      }
                    }
                    n116 = flat-sequence {
                      tunnel: w187 -> [w194]
                      tunnel: [w201] -> w188
                      frame #0 {
                        n117 = while {
                          tunnel: w194 -> [w195]
                          stop <- w196 stop-if-true
                          n118 = call "Turn Angle.vi"("setpoint"=w195) -> ("In Range?"=w196:bool)  [unwired: 10 in]
                        }
                      }
                      frame #1 {
                        w197 = 0.0
                        n119 = global read "Robot Values.vi" "Robot Values"() -> (w198:T10)
                        n120 = Bundle By Name(cluster=w198, "Drive Motors.Left Motor Value"=w197, "Drive Motors.Right Motor Value"=w197) -> (w199:T10)
                        n121 = Wait (ms)(milliseconds to wait=u32 500) -> ()  [unwired: 1 out]
                        n122 = global write "Robot Values.vi" "Robot Values"(w199) -> ()
                      }
                      frame #2 {
                        n123 = global read "Robot Values.vi" "Robot Values"() -> (w205:T10)
                        n124 = Unbundle By Name(w205) -> ("Sensors.Gyro Angle"=w204:dbl)
                        n125 = In Range and Coerce(upper limit=182.0, x=w204, lower limit=178.0 ("x")) -> (In Range?=w201:bool)  [unwired: 1 out]
                      }
                    }
                    n126 = disable-structure shown="Enabled" {
                      disable-tunnel: w190 -> [w207 w208]
                      disable-tunnel: [w206 _] -> _
                      disable-tunnel: [_ w208] -> w187
                      frame Disabled {
                        n127 = call "Turn Angle.vi"("setpoint"=w207) -> ("In Range?"=w206:bool)  [unwired: 10 in]
                      }
                      frame Enabled {
                      }
                    }
                    n128 = Select(t=AutoStatesTypeDef."Line up to shoot" ("Defense"), s=w188, f=w193) -> (s? t:f=w192:T2)
                  }
                  frame "Line up to shoot" {
                    n129 = call "Align to Shoot.vi"() -> ("Stop?"=w216:bool, "Aligned?"=w220:bool)  [unwired: 10 in]
                    n130 = Select(t=AutoStatesTypeDef."Stop" ("Defense"), s=w216, f=w219) -> (s? t:f=w218:T2)
                    n131 = Select(t=AutoStatesTypeDef."Shoot" ("Defense"), s=w220, f=w218) -> (s? t:f=w222:T2)
                  }
                  frame "Initialize" {
                    n132 = flat-sequence {
                      tunnel: [AutoStatesTypeDef."Drive to defense" ("t")] -> w223
                      frame #0 {
                        n133 = global read "Robot Values.vi" "Robot Values"() -> (w226:T10)
                        n134 = Bundle By Name(cluster=w226, "Sensors.Reset Gyro?"=TRUE ("Arms.Initialize Arm Position?")) -> (w225:T10)
                        n135 = global write "Robot Values.vi" "Robot Values"(w225) -> ()
                      }
                      frame #1 {
                        w227 = FALSE ("Arms.Initialize Arm Position?")
                        n136 = global read "Robot Global.vi" "Global Refs"() -> (w231:T11)
                        n137 = Unbundle By Name(w231) -> ("Sensor.Left Drive EncoderDevRef"=w233:T26, "Sensor.Right Drive EncoderDevRef"=w232:T26)
                        n138 = call <vilib>:"WPI_EncoderReset.vi"("EncoderDevRef"=w233) -> ("EncoderDevRef"=w230:T26)  [unwired: 9 in, 1 out]
                        n139 = call <vilib>:"WPI_EncoderReset.vi"("EncoderDevRef"=w232) -> ("EncoderDevRef"=w229:T26)  [unwired: 9 in, 1 out]
                        n140 = Bundle By Name(cluster=w231, "Sensor.Left Drive EncoderDevRef"=w230, "Sensor.Right Drive EncoderDevRef"=w229) -> (w228:T11)
                        n141 = global read "Robot Values.vi" "Robot Values"() -> (w236:T10)
                        n142 = Bundle By Name(cluster=w236, "Arms.Initialize Arm Position?"=w227, "Sensors.Reset Gyro?"=w227, "Acquisition and Scoring.Acquiring?"=w227) -> (w237:T10)
                        n143 = Wait (ms)(milliseconds to wait=u32 25) -> ()  [unwired: 1 out]
                        n144 = global write "Robot Values.vi" "Robot Values"(w237) -> ()
                        n145 = global write "Robot Global.vi" "Global Refs"(w228) -> ()
                      }
                    }
                  }
                  frame "Lower Arms" {
                    n146 = flat-sequence {
                      tunnel: [AutoStatesTypeDef."Raise Arms" ("t")] -> w238
                      frame #0 {
                        n147 = while {
                          stop <- w244 stop-if-true
                          n148 = global read "Robot Values.vi" "Robot Values"() -> (w246:T10)
                          n149 = First Call?() -> (First Call?: T/F=w243:bool)
                          n150 = Unbundle By Name(w246) -> ("Arms.Left Arm Lower Limit"=w245:bool)
                          n151 = call "1038 Timer.vi"("Reset?"=w243, "Time Target"=1.5) -> ("Done?"=w241:bool)  [unwired: 9 in]
                          n152 = global read "Robot Values.vi" "Robot Values"() -> (w248:T10)
                          n153 = Bundle By Name(cluster=w248, "Arms.Initialize Arm Position?"=TRUE) -> (w247:T10)
                          n154 = Wait (ms)(milliseconds to wait=u32 25) -> ()  [unwired: 1 out]
                          n155 = global write "Robot Values.vi" "Robot Values"(w247) -> ()
                          n156 = Or(x=w241, y=w245) -> (x .or. y?=w244:bool)
                        }
                      }
                      frame #1 {
                        n157 = global read "Robot Global.vi" "Global Refs"() -> (w255:T11)
                        n158 = Unbundle By Name(w255) -> ("Sensor.Left Drive EncoderDevRef"=w257:T26, "Sensor.Right Drive EncoderDevRef"=w256:T26)
                        n159 = global read "Robot Values.vi" "Robot Values"() -> (w251:T10)
                        n160 = Bundle By Name(cluster=w251, "Arms.Initialize Arm Position?"=FALSE) -> (w250:T10)
                        n161 = global write "Robot Values.vi" "Robot Values"(w250) -> ()
                        n162 = call <vilib>:"WPI_EncoderReset.vi"("EncoderDevRef"=w257) -> ("EncoderDevRef"=w254:T26)  [unwired: 9 in, 1 out]
                        n163 = call <vilib>:"WPI_EncoderReset.vi"("EncoderDevRef"=w256) -> ("EncoderDevRef"=w253:T26)  [unwired: 9 in, 1 out]
                        n164 = Wait (ms)(milliseconds to wait=u32 5) -> ()  [unwired: 1 out]
                        n165 = Bundle By Name(cluster=w255, "Sensor.Left Drive EncoderDevRef"=w254, "Sensor.Right Drive EncoderDevRef"=w253) -> (w252:T11)
                        n166 = global write "Robot Global.vi" "Global Refs"(w252) -> ()
                      }
                    }
                  }
                  frame "Raise Arms" {
                    n167 = flat-sequence {
                      tunnel: [AutoStatesTypeDef."Cross defense" ("t")] -> w260
                      frame #0 {
                        n168 = while {
                          stop <- w261 stop-if-true
                          n169 = call "Drive Straight Gyro.vi"("Distance to travel"=100.0) -> ("In Range?"=w261:bool)  [unwired: 10 in]
                        }
                      }
                      frame #1 {
                        n170 = while {
                          stop <- w265 stop-if-true
                          w266 = 0.0
                          n171 = First Call?() -> (First Call?: T/F=w272:bool)
                          n172 = call "1038 Timer.vi"("Reset?"=w272, "Time Target"=0.25) -> ("Done?"=w265:bool)  [unwired: 9 in]
                          n173 = Select(t=0.0, s=w265, f=-1.0) -> (s? t:f=w273:dbl)
                          n174 = global read "Robot Values.vi" "Robot Values"() -> (w267:T10)
                          n175 = Bundle By Name(cluster=w267, "Drive Motors.Left Motor Value"=w266, "Drive Motors.Right Motor Value"=w266) -> (w268:T10)
                          n176 = global read "Robot Values.vi" "Robot Values"() -> (w263:T10)
                          n177 = Bundle By Name(cluster=w263, "Arms.Desired Arm Position"=w273) -> (w264:T10)
                          n178 = global write "Robot Values.vi" "Robot Values"(w268) -> ()
                          n179 = global write "Robot Values.vi" "Robot Values"(w264) -> ()
                        }
                      }
                      frame #2 {
                        n180 = global read "Robot Global.vi" "Global Refs"() -> (w278:T11)
                        n181 = Unbundle By Name(w278) -> ("Sensor.Left Drive EncoderDevRef"=w280:T26, "Sensor.Right Drive EncoderDevRef"=w279:T26)
                        n182 = Wait (ms)(milliseconds to wait=u32 5) -> ()  [unwired: 1 out]
                        n183 = call <vilib>:"WPI_EncoderReset.vi"("EncoderDevRef"=w280) -> ("EncoderDevRef"=w277:T26)  [unwired: 9 in, 1 out]
                        n184 = call <vilib>:"WPI_EncoderReset.vi"("EncoderDevRef"=w279) -> ("EncoderDevRef"=w276:T26)  [unwired: 9 in, 1 out]
                        n185 = Bundle By Name(cluster=w278, "Sensor.Left Drive EncoderDevRef"=w277, "Sensor.Right Drive EncoderDevRef"=w276) -> (w275:T11)
                        n186 = global write "Robot Global.vi" "Global Refs"(w275) -> ()
                      }
                    }
                  }
                }
              }
            }
          }
          frame "CDF" {
            n187 = case shown="\"Cross defense\"" w284 {
              selector: w284 -> [_ w318 w340 w375 _ _ w384 w398 w433 _ _]
              tunnel: [w286 w319 w341 w374 AutoStatesTypeDef."Drive to goal" ("Defense") AutoStatesTypeDef."Stop" ("Defense") w387 w397 w434 w435 w452] -> w282
              tunnel: w283 -> [w288 w316 w339 _ _ _ _ w395 _ _ _]
              frame "Drive to goal" {
                (unwired) AutoStatesTypeDef."Turn towards goal" ("t")
                n188 = case shown="\"Second\"" w288 {
                  tunnel: [0.0 ("setpoint") w308 w309 w312 w313] -> w285
                  frame "First", Default {
                  }
                  frame "Second" {
                    n189 = local read "Pos 2 Drive"() -> (w308:dbl)
                  }
                  frame "Third" {
                    n190 = disable-structure shown="Enabled" {
                      disable-tunnel: [w310 -150.0 ("Pos 3 Drive")] -> w309
                      frame Disabled {
                        n191 = local read "Pos 3 Drive"() -> (w310:dbl)
                      }
                      frame Enabled {
                      }
                    }
                  }
                  frame "Fourth" {
                    n192 = local read "Pos 4 Drive"() -> (w312:dbl)
                  }
                  frame "Fifth" {
                    n193 = local read "Pos 5 Drive"() -> (w313:dbl)
                  }
                }
                n194 = flat-sequence {
                  tunnel: [w297] -> w287
                  tunnel: w285 -> [w296]
                  tunnel: [w306] -> w286
                  tunnel: w287 -> [w306]
                  frame #0 {
                    n195 = global read "Robot Global.vi" "Global Refs"() -> (w293:T11)
                    n196 = Unbundle By Name(w293) -> ("Sensor.Left Drive EncoderDevRef"=w295:T26, "Sensor.Right Drive EncoderDevRef"=w294:T26)
                    n197 = call <vilib>:"WPI_EncoderReset.vi"("EncoderDevRef"=w295) -> ("EncoderDevRef"=w292:T26)  [unwired: 9 in, 1 out]
                    n198 = call <vilib>:"WPI_EncoderReset.vi"("EncoderDevRef"=w294) -> ("EncoderDevRef"=w291:T26)  [unwired: 9 in, 1 out]
                    n199 = Wait (ms)(milliseconds to wait=u32 25) -> ()  [unwired: 1 out]
                    n200 = Bundle By Name(cluster=w293, "Sensor.Left Drive EncoderDevRef"=w292, "Sensor.Right Drive EncoderDevRef"=w291) -> (w290:T11)
                    n201 = global write "Robot Global.vi" "Global Refs"(w290) -> ()
                  }
                  frame #1 {
                    n202 = while {
                      tunnel: [w299] -> w297
                      tunnel: w296 -> [w298]
                      stop <- w301 stop-if-true
                      n203 = call "Drive Straight Gyro.vi"("Distance to travel"=w298) -> ("In Range?"=w301:bool)  [unwired: 10 in]
                      n204 = Select(t=AutoStatesTypeDef."Turn towards goal" ("Defense"), s=w301, f=AutoStatesTypeDef."Drive to goal") -> (s? t:f=w299:T2)
                      n205 = call "Auton Reaquire.vi"() -> ()  [unwired: 12 in]
                    }
                  }
                  frame #2 {
                    w303 = 0.0
                    n206 = global read "Robot Values.vi" "Robot Values"() -> (w304:T10)
                    n207 = Bundle By Name(cluster=w304, "Drive Motors.Left Motor Value"=w303, "Drive Motors.Right Motor Value"=w303) -> (w305:T10)
                    n208 = global write "Robot Values.vi" "Robot Values"(w305) -> ()
                  }
                }
              }
              frame "Turn towards goal" {
                # "Turns the robot to face toward the goal"
                n209 = case shown="\"Second\"" w316 {
                  tunnel: [0.0 ("setpoint") w335 w336 w337 w338] -> w315
                  frame "First", Default {
                  }
                  frame "Second" {
                    n210 = local read "Pos 2 Turn"() -> (w335:dbl)
                  }
                  frame "Third" {
                    n211 = local read "Pos 3 Turn"() -> (w336:dbl)
                  }
                  frame "Fourth" {
                    n212 = local read "Pos 4 Turn"() -> (w337:dbl)
                  }
                  frame "Fifth" {
                    n213 = local read "Pos 5 Turn"() -> (w338:dbl)
                  }
                }
                n214 = flat-sequence {
                  tunnel: w315 -> [w320]
                  tunnel: [w331] -> w314
                  tunnel: w315 -> [w329]
                  frame #0 {
                    n215 = while {
                      tunnel: w320 -> [w321]
                      stop <- w322 stop-if-true
                      n216 = call "Turn Angle.vi"("setpoint"=w321) -> ("In Range?"=w322:bool)  [unwired: 10 in]
                    }
                  }
                  frame #1 {
                    w323 = 0.0
                    n217 = global read "Robot Values.vi" "Robot Values"() -> (w324:T10)
                    n218 = Bundle By Name(cluster=w324, "Drive Motors.Left Motor Value"=w323, "Drive Motors.Right Motor Value"=w323) -> (w325:T10)
                    n219 = Wait (ms)(milliseconds to wait=u32 500) -> ()  [unwired: 1 out]
                    n220 = global write "Robot Values.vi" "Robot Values"(w325) -> ()
                  }
                  frame #2 {
                    w330 = 2.0
                    n221 = global read "Robot Values.vi" "Robot Values"() -> (w333:T10)
                    n222 = Unbundle By Name(w333) -> ("Sensors.Gyro Angle"=w332:dbl)
                    n223 = Add(x=w329, y=w330) -> (x+y=w328:dbl)
                    n224 = Subtract(x=w329, y=w330) -> (x-y=w327:dbl)
                    n225 = In Range and Coerce(upper limit=w328, x=w332, lower limit=w327) -> (In Range?=w331:bool)  [unwired: 1 out]
                  }
                }
                n226 = Select(t=AutoStatesTypeDef."Line up to shoot" ("Defense"), s=w314, f=w318) -> (s? t:f=w319:T2)
              }
              frame "Cross defense" {
                n227 = disable-structure shown="Enabled" {
                  disable-tunnel: [w346 w357] -> w341
                  disable-tunnel: w340 -> [w344 w358]
                  disable-tunnel: w339 -> [_ w352]
                  frame Disabled {
                    # "Checks for rise and fall of accelerometer to verify robot has croseed the defense"
                    # "Drives robot forward over defense"
                    # "encoder counts"
                    n228 = call "Check Lowbar Cross.vi"() -> ("Cross"=w343:bool)  [unwired: 11 in]
                    n229 = call "Drive Straight Gyro.vi"("Distance to travel"=-1200.0) -> ()  [unwired: 10 in, 1 out]
                    n230 = Select(t=AutoStatesTypeDef."Stop" ("Defense"), s=w343, f=w344) -> (s? t:f=w346:T2)
                  }
                  frame Enabled {
                    # "Shouldn't ever be in this case in low bar auton"
                    n231 = global read "Robot Values.vi" "Robot Values"() -> (w363:T10)
                    n232 = Equal?(x=w352, y=T9."First") -> (x = y?=w347:bool)
                    n233 = Unbundle By Name(w363) -> ("Drive Motors.Left Motor Encoder"=w362:dbl)
                    n234 = Less?(x=w362, y=90.0) -> (x < y?=w356:bool)
                    n235 = Select(t=AutoStatesTypeDef."Stop", s=w347, f=AutoStatesTypeDef."Align robot" ("t")) -> (s? t:f=w350:T2)
                    n236 = call "Drive Straight Gyro.vi"("output range"=cluster{"output high":dbl, "output low":dbl} {"output high"=0.8, "output low"=-0.8}, "Distance to travel"=800.0) -> ("In Range?"=w359:bool)  [unwired: 9 in]
                    n237 = case shown="False" w356 {
                      selector: w356 -> [w371 w373]
                      tunnel: [w371 w373] -> w355
                      tunnel: [w365 0.0] -> w354
                      frame False {
                        n238 = First Call?() -> (First Call?: T/F=w370:bool)
                        n239 = call "1038 Timer.vi"("Reset?"=w370, "Time Target"=3.0) -> ("Done?"=w368:bool)  [unwired: 9 in]
                        n240 = Select(t=0.0, s=w368, f=-1.0) -> (s? t:f=w365:dbl)
                      }
                      frame True {
                      }
                    }
                    n241 = Select(t=w350, s=w359, f=w358) -> (s? t:f=w357:T2)
                    n242 = call "Auton Reaquire.vi"() -> ()  [unwired: 12 in]
                    n243 = Bundle By Name(cluster=w363, "Arms.Initialize Arm Position?"=w355, "Arms.Desired Arm Position"=w354) -> (w364:T10)
                    n244 = global write "Robot Values.vi" "Robot Values"(w364) -> ()
                  }
                }
              }
              frame "Shoot" {
                # "Prep wheels for a set time before shooting.\nshoot. switch to stop case after 1 second"
                n245 = call "Autonomous shoot.vi"() -> ("Shot?"=w376:bool)  [unwired: 11 in]
                n246 = Select(t=AutoStatesTypeDef."Stop" ("Defense"), s=w376, f=w375) -> (s? t:f=w374:T2)
              }
              frame "Retreat" {
                # "Maybe move wheels back?"
              }
              frame "Stop", Default {
                w379 = FALSE ("Arms.Initialize Arm Position?")
                w380 = 0.0
                # "Close Stuff"
                n247 = global read "Robot Values.vi" "Robot Values"() -> (w382:T10)
                n248 = Bundle By Name(cluster=w382, "Drive Motors.Left Motor Value"=w380, "Drive Motors.Right Motor Value"=w380, "Arms.Initialize Arm Position?"=w379, "Acquisition and Scoring.Prep Wheels"=w379, "Acquisition and Scoring.Shoot"=w379) -> (w381:T10)
                n249 = global write "Robot Values.vi" "Robot Values"(w381) -> ()
              }
              frame "Drive to defense" {
                # "Will drive straight until setpoint is reached. Need to add proper setpoint"
                n250 = call "Drive Straight Gyro.vi"("Distance to travel"=245.0) -> ("In Range?"=w385:bool)  [unwired: 10 in]
                n251 = Select(t=AutoStatesTypeDef."Lower Arms" ("Defense"), s=w385, f=w384) -> (s? t:f=w387:T2)
              }
              frame "Align robot" {
                # "Turns the robot around to face toward the goal"
                n252 = case shown="\"First\", Default" w395 {
                  tunnel: [0.0 ("setpoint") w418 w419 w422 w423] -> w396
                  tunnel: [TRUE _ _ _ _] -> w389
                  frame "First", Default {
                  }
                  frame "Second" {
                    n253 = local read "Pos 2 Align"() -> (w418:dbl)
                  }
                  frame "Third" {
                    n254 = disable-structure shown="Enabled" {
                      disable-tunnel: [w420 180.0 ("Pos 3 Align")] -> w419
                      frame Enabled {
                        n255 = local read "Pos 3 Align"() -> (w420:dbl)
                      }
                      frame Disabled {
                      }
                    }
                  }
                  frame "Fourth" {
                    n256 = local read "Pos 4 Align"() -> (w422:dbl)
                  }
                  frame "Fifth" {
                    n257 = local read "Pos 5 Align"() -> (w423:dbl)
                  }
                }
                n258 = flat-sequence {
                  tunnel: w393 -> [w399]
                  tunnel: [w410] -> w394
                  tunnel: w393 -> [w408]
                  frame #0 {
                    n259 = while {
                      tunnel: w399 -> [w400]
                      stop <- w401 stop-if-true
                      n260 = call "Turn Angle.vi"("setpoint"=w400) -> ("In Range?"=w401:bool)  [unwired: 10 in]
                    }
                  }
                  frame #1 {
                    w402 = 0.0
                    n261 = global read "Robot Values.vi" "Robot Values"() -> (w403:T10)
                    n262 = Bundle By Name(cluster=w403, "Drive Motors.Left Motor Value"=w402, "Drive Motors.Right Motor Value"=w402) -> (w404:T10)
                    n263 = Wait (ms)(milliseconds to wait=u32 500) -> ()  [unwired: 1 out]
                    n264 = global write "Robot Values.vi" "Robot Values"(w404) -> ()
                  }
                  frame #2 {
                    w409 = 2.0
                    n265 = global read "Robot Values.vi" "Robot Values"() -> (w412:T10)
                    n266 = Unbundle By Name(w412) -> ("Sensors.Gyro Angle"=w411:dbl)
                    n267 = Add(x=w408, y=w409) -> (x+y=w407:dbl)
                    n268 = Subtract(x=w408, y=w409) -> (x-y=w406:dbl)
                    n269 = In Range and Coerce(upper limit=w407, x=w411, lower limit=w406) -> (In Range?=w410:bool)  [unwired: 1 out]
                  }
                }
                n270 = disable-structure shown="Enabled" {
                  disable-tunnel: w396 -> [w414 w415]
                  disable-tunnel: [w413 _] -> _
                  disable-tunnel: [_ w415] -> w393
                  frame Disabled {
                    n271 = call "Turn Angle.vi"("setpoint"=w414) -> ("In Range?"=w413:bool)  [unwired: 10 in]
                  }
                  frame Enabled {
                  }
                }
                n272 = Select(t=AutoStatesTypeDef."Stop", s=w389, f=AutoStatesTypeDef."Drive to goal" ("Defense")) -> (s? t:f=w391:T2)
                n273 = Select(t=w391, s=w394, f=w398) -> (s? t:f=w397:T2)
              }
              frame "Line up to shoot" {
                w428 = AutoStatesTypeDef."Stop" ("Defense")
                n274 = call-poly <vilib>:"NT Read Value.vi"("Default Value"=TRUE, "Name"="Auton Shoot") -> ("Boolean"=w424:bool)  [unwired: 8 in, 1 out]
                n275 = call "Align to Shoot.vi"() -> ("Stop?"=w430:bool, "Aligned?"=w432:bool)  [unwired: 10 in]
                n276 = Select(t=AutoStatesTypeDef."Shoot" ("Defense"), s=w424, f=w428) -> (s? t:f=w427:T2)
                n277 = Select(t=w428, s=w430, f=w433) -> (s? t:f=w431:T2)
                n278 = Select(t=w427, s=w432, f=w431) -> (s? t:f=w434:T2)
              }
              frame "Initialize" {
                n279 = flat-sequence {
                  tunnel: [AutoStatesTypeDef."Drive to defense" ("t")] -> w435
                  frame #0 {
                    n280 = global read "Robot Values.vi" "Robot Values"() -> (w440:T10)
                    n281 = Bundle By Name(cluster=w440, "Arms.Initialize Arm Position?"=FALSE, "Sensors.Reset Gyro?"=TRUE ("Arms.Initialize Arm Position?")) -> (w439:T10)
                    n282 = Wait (ms)(milliseconds to wait=u32 25) -> ()  [unwired: 1 out]
                    n283 = global write "Robot Values.vi" "Robot Values"(w439) -> ()
                  }
                  frame #1 {
                    w441 = FALSE ("Arms.Initialize Arm Position?")
                    n284 = global read "Robot Global.vi" "Global Refs"() -> (w445:T11)
                    n285 = Unbundle By Name(w445) -> ("Sensor.Left Drive EncoderDevRef"=w447:T26, "Sensor.Right Drive EncoderDevRef"=w446:T26)
                    n286 = call <vilib>:"WPI_EncoderReset.vi"("EncoderDevRef"=w447) -> ("EncoderDevRef"=w444:T26)  [unwired: 9 in, 1 out]
                    n287 = call <vilib>:"WPI_EncoderReset.vi"("EncoderDevRef"=w446) -> ("EncoderDevRef"=w443:T26)  [unwired: 9 in, 1 out]
                    n288 = Bundle By Name(cluster=w445, "Sensor.Left Drive EncoderDevRef"=w444, "Sensor.Right Drive EncoderDevRef"=w443) -> (w442:T11)
                    n289 = global read "Robot Values.vi" "Robot Values"() -> (w450:T10)
                    n290 = Bundle By Name(cluster=w450, "Arms.Initialize Arm Position?"=w441, "Sensors.Reset Gyro?"=w441, "Acquisition and Scoring.Acquiring?"=w441) -> (w451:T10)
                    n291 = Wait (ms)(milliseconds to wait=u32 25) -> ()  [unwired: 1 out]
                    n292 = global write "Robot Values.vi" "Robot Values"(w451) -> ()
                    n293 = global write "Robot Global.vi" "Global Refs"(w442) -> ()
                  }
                }
              }
              frame "Lower Arms" {
                n294 = flat-sequence {
                  tunnel: [AutoStatesTypeDef."Cross defense" ("t")] -> w452
                  frame #0 {
                    n295 = while {
                      stop <- w459 stop-if-true
                      n296 = disable-structure shown="Enabled" {
                        disable-tunnel: [0.2 0.0] -> w453
                        frame Disabled {
                        }
                        frame Enabled {
                        }
                      }
                      n297 = global read "Robot Values.vi" "Robot Values"() -> (w461:T10)
                      n298 = First Call?() -> (First Call?: T/F=w458:bool)
                      n299 = Unbundle By Name(w461) -> ("Arms.Left Arm Lower Limit"=w460:bool)
                      n300 = call "1038 Timer.vi"("Reset?"=w458, "Time Target"=1.8) -> ("Done?"=w456:bool)  [unwired: 9 in]
                      n301 = global read "Robot Values.vi" "Robot Values"() -> (w463:T10)
                      n302 = Bundle By Name(cluster=w463, "Arms.Initialize Arm Position?"=TRUE, "Drive Motors.Left Motor Value"=w453, "Drive Motors.Right Motor Value"=w453) -> (w462:T10)
                      n303 = Wait (ms)(milliseconds to wait=u32 25) -> ()  [unwired: 1 out]
                      n304 = global write "Robot Values.vi" "Robot Values"(w462) -> ()
                      n305 = Or(x=w456, y=w460) -> (x .or. y?=w459:bool)
                    }
                  }
                  frame #1 {
                    n306 = global read "Robot Global.vi" "Global Refs"() -> (w469:T11)
                    n307 = Unbundle By Name(w469) -> ("Sensor.Left Drive EncoderDevRef"=w471:T26, "Sensor.Right Drive EncoderDevRef"=w470:T26)
                    n308 = call <vilib>:"WPI_EncoderReset.vi"("EncoderDevRef"=w471) -> ("EncoderDevRef"=w468:T26)  [unwired: 9 in, 1 out]
                    n309 = call <vilib>:"WPI_EncoderReset.vi"("EncoderDevRef"=w470) -> ("EncoderDevRef"=w467:T26)  [unwired: 9 in, 1 out]
                    n310 = Wait (ms)(milliseconds to wait=u32 5) -> ()  [unwired: 1 out]
                    n311 = Bundle By Name(cluster=w469, "Sensor.Left Drive EncoderDevRef"=w468, "Sensor.Right Drive EncoderDevRef"=w467) -> (w466:T11)
                    n312 = global write "Robot Global.vi" "Global Refs"(w466) -> ()
                  }
                }
              }
            }
          }
          frame "Moat" {
            n313 = case shown="\"Initialize\"" w476 {
              selector: w476 -> [w480 w491 w499 w509 _ _ w521 w531 w540 _]
              tunnel: [w482 w493 w500 w508 AutoStatesTypeDef."Drive to goal" ("Defense") AutoStatesTypeDef."Stop" ("Defense") w524 w530 w543 w544] -> w474
              tunnel: w475 -> [w478 w489 _ _ _ _ _ w526 _ _]
              frame "Drive to goal" {
                n314 = case shown="\"Fifth\"" w478 {
                  tunnel: [0.0 ("setpoint") w484 w485 w486 w487] -> w477
                  frame "First", Default {
                  }
                  frame "Second" {
                    n315 = local read "Pos 2 Drive"() -> (w484:dbl)
                  }
                  frame "Third" {
                    n316 = local read "Pos 3 Drive"() -> (w485:dbl)
                  }
                  frame "Fourth" {
                    n317 = local read "Pos 4 Drive"() -> (w486:dbl)
                  }
                  frame "Fifth" {
                    n318 = local read "Pos 5 Drive"() -> (w487:dbl)
                  }
                }
                n319 = call "Drive Straight Gyro.vi"("Distance to travel"=w477) -> ("In Range?"=w479:bool)  [unwired: 10 in]
                n320 = Select(t=AutoStatesTypeDef."Turn towards goal", s=w479, f=w480) -> (s? t:f=w482:T2)
              }
              frame "Turn towards goal" {
                # "Turns the robot to face toward the goal"
                n321 = case shown="\"Fifth\"" w489 {
                  tunnel: [0.0 ("setpoint") w495 w496 w497 w498] -> w488
                  frame "First", Default {
                  }
                  frame "Second" {
                    n322 = local read "Pos 2 Turn"() -> (w495:dbl)
                  }
                  frame "Third" {
                    n323 = local read "Pos 3 Turn"() -> (w496:dbl)
                  }
                  frame "Fourth" {
                    n324 = local read "Pos 4 Turn"() -> (w497:dbl)
                  }
                  frame "Fifth" {
                    n325 = local read "Pos 5 Turn"() -> (w498:dbl)
                  }
                }
                n326 = call "Turn Angle.vi"("setpoint"=w488) -> ("In Range?"=w492:bool)  [unwired: 10 in]
                n327 = Select(t=AutoStatesTypeDef."Line up to shoot" ("Defense"), s=w492, f=w491) -> (s? t:f=w493:T2)
              }
              frame "Cross defense" {
                n328 = disable-structure shown="Enabled" {
                  disable-tunnel: [w505 AutoStatesTypeDef."Stop" ("Defense")] -> w500
                  disable-tunnel: w499 -> [w503 _]
                  frame Disabled {
                    # "Checks for rise and fall of accelerometer to verify robot has croseed the defense"
                    # "Drives robot forward over defense"
                    # "encoder counts"
                    n329 = call "Check Lowbar Cross.vi"() -> ("Cross"=w502:bool)  [unwired: 11 in]
                    n330 = call "Drive Straight Gyro.vi"("Distance to travel"=-1200.0) -> ()  [unwired: 10 in, 1 out]
                    n331 = Select(t=AutoStatesTypeDef."Stop" ("Defense"), s=w502, f=w503) -> (s? t:f=w505:T2)
                  }
                  frame Enabled {
                    # "Shouldn't ever be in this case in low bar auton"
                  }
                }
              }
              frame "Shoot" {
                # "Prep wheels for a set time before shooting.\nshoot. switch to stop case after 1 second"
                n332 = call "Autonomous shoot.vi"() -> ("Shot?"=w511:bool)  [unwired: 11 in]
                n333 = call "1038 Timer.vi"("Reset?"=w511, "Time Target"=2.0) -> ("Done?"=w507:bool)  [unwired: 9 in]
                n334 = Select(t=AutoStatesTypeDef."Stop" ("Defense"), s=w507, f=w509) -> (s? t:f=w508:T2)
              }
              frame "Retreat" {
                # "Maybe move wheels back?"
              }
              frame "Stop", Default {
                w514 = FALSE ("Arms.Initialize Arm Position?")
                w515 = 0.0
                # "Close Stuff"
                n335 = global read "Robot Values.vi" "Robot Values"() -> (w517:T10)
                n336 = Bundle By Name(cluster=w517, "Drive Motors.Left Motor Value"=w515, "Drive Motors.Right Motor Value"=w515, "Arms.Initialize Arm Position?"=w514, "Acquisition and Scoring.Prep Wheels"=w514, "Acquisition and Scoring.Shoot"=w514) -> (w516:T10)
                n337 = global write "Robot Values.vi" "Robot Values"(w516) -> ()
              }
              frame "Drive to defense" {
                # "Will drive straight until setpoint is reached. Need to add proper setpoint"
                n338 = call "Drive Straight Gyro.vi"("PID gains"="PID gains 5", "output range"=cluster{"output high":dbl, "output low":dbl} {"output high"=1.0, "output low"=-1.0}, "Distance to travel"=-1000.0) -> ("In Range?"=w522:bool)  [unwired: 8 in]
                n339 = Select(t=AutoStatesTypeDef."Align robot" ("Defense"), s=w522, f=w521) -> (s? t:f=w524:T2)
              }
              frame "Align robot" {
                # "Returns robot to staight position after crossing defense"
                n340 = case shown="\"Fifth\"" w526 {
                  tunnel: [0.0 ("setpoint") w533 w534 w535 w536] -> w528
                  frame "First", Default {
                  }
                  frame "Second" {
                    n341 = local read "Pos 2 Align"() -> (w533:dbl)
                  }
                  frame "Third" {
                    n342 = local read "Pos 3 Align"() -> (w534:dbl)
                  }
                  frame "Fourth" {
                    n343 = local read "Pos 4 Align"() -> (w535:dbl)
                  }
                  frame "Fifth" {
                    n344 = local read "Pos 5 Align"() -> (w536:dbl)
                  }
                }
                n345 = call "Turn Angle.vi"("setpoint"=w528) -> ("In Range?"=w527:bool)  [unwired: 10 in]
                n346 = Select(t=AutoStatesTypeDef."Drive to goal" ("Defense"), s=w527, f=w531) -> (s? t:f=w530:T2)
              }
              frame "Line up to shoot" {
                n347 = call "Align to Shoot.vi"() -> ("Stop?"=w537:bool, "Aligned?"=w541:bool)  [unwired: 10 in]
                n348 = Select(t=AutoStatesTypeDef."Stop" ("Defense"), s=w537, f=w540) -> (s? t:f=w539:T2)
                n349 = Select(t=AutoStatesTypeDef."Shoot" ("Defense"), s=w541, f=w539) -> (s? t:f=w543:T2)
              }
              frame "Initialize" {
                n350 = flat-sequence {
                  tunnel: [AutoStatesTypeDef."Drive to defense" ("t")] -> w544
                  frame #0 {
                    n351 = while {
                      stop <- w548 stop-if-true
                      n352 = global read "Robot Values.vi" "Robot Values"() -> (w551:T10)
                      n353 = Unbundle By Name(w551) -> ("Arms.Left Arm Lower Limit"=w549:bool)
                      n354 = First Call?() -> (First Call?: T/F=w547:bool)
                      n355 = global read "Robot Values.vi" "Robot Values"() -> (w553:T10)
                      n356 = Bundle By Name(cluster=w553, "Sensors.Reset Gyro?"=TRUE ("Arms.Initialize Arm Position?")) -> (w552:T10)
                      n357 = call "1038 Timer.vi"("Reset?"=w547, "Time Target"=5.0) -> ("Done?"=w545:bool)  [unwired: 9 in]
                      n358 = global write "Robot Values.vi" "Robot Values"(w552) -> ()
                      n359 = Or(x=w545, y=w549) -> (x .or. y?=w548:bool)
                    }
                  }
                  frame #1 {
                    w557 = FALSE ("Arms.Initialize Arm Position?")
                    n360 = global read "Robot Values.vi" "Robot Values"() -> (w555:T10)
                    n361 = Bundle By Name(cluster=w555, "Arms.Initialize Arm Position?"=w557, "Sensors.Reset Gyro?"=w557) -> (w556:T10)
                    n362 = global write "Robot Values.vi" "Robot Values"(w556) -> ()
                  }
                }
              }
            }
          }
          frame "Ramparts" {
            n363 = case shown="\"Initialize\"" w560 {
              selector: w560 -> [w564 w575 w583 w593 _ _ w605 w615 w624 _]
              tunnel: [w566 w577 w584 w592 AutoStatesTypeDef."Drive to goal" ("Defense") AutoStatesTypeDef."Stop" ("Defense") w608 w614 w627 w628] -> w558
              tunnel: w559 -> [w562 w573 _ _ _ _ _ w610 _ _]
              frame "Drive to goal" {
                n364 = case shown="\"Fifth\"" w562 {
                  tunnel: [0.0 ("setpoint") w568 w569 w570 w571] -> w561
                  frame "First", Default {
                  }
                  frame "Second" {
                    n365 = local read "Pos 2 Drive"() -> (w568:dbl)
                  }
                  frame "Third" {
                    n366 = local read "Pos 3 Drive"() -> (w569:dbl)
                  }
                  frame "Fourth" {
                    n367 = local read "Pos 4 Drive"() -> (w570:dbl)
                  }
                  frame "Fifth" {
                    n368 = local read "Pos 5 Drive"() -> (w571:dbl)
                  }
                }
                n369 = call "Drive Straight Gyro.vi"("Distance to travel"=w561) -> ("In Range?"=w563:bool)  [unwired: 10 in]
                n370 = Select(t=AutoStatesTypeDef."Turn towards goal", s=w563, f=w564) -> (s? t:f=w566:T2)
              }
              frame "Turn towards goal" {
                # "Turns the robot to face toward the goal"
                n371 = case shown="\"Fifth\"" w573 {
                  tunnel: [0.0 ("setpoint") w579 w580 w581 w582] -> w572
                  frame "First", Default {
                  }
                  frame "Second" {
                    n372 = local read "Pos 2 Turn"() -> (w579:dbl)
                  }
                  frame "Third" {
                    n373 = local read "Pos 3 Turn"() -> (w580:dbl)
                  }
                  frame "Fourth" {
                    n374 = local read "Pos 4 Turn"() -> (w581:dbl)
                  }
                  frame "Fifth" {
                    n375 = local read "Pos 5 Turn"() -> (w582:dbl)
                  }
                }
                n376 = call "Turn Angle.vi"("setpoint"=w572) -> ("In Range?"=w576:bool)  [unwired: 10 in]
                n377 = Select(t=AutoStatesTypeDef."Line up to shoot" ("Defense"), s=w576, f=w575) -> (s? t:f=w577:T2)
              }
              frame "Cross defense" {
                n378 = disable-structure shown="Enabled" {
                  disable-tunnel: [w589 AutoStatesTypeDef."Stop" ("Defense")] -> w584
                  disable-tunnel: w583 -> [w587 _]
                  frame Disabled {
                    # "Checks for rise and fall of accelerometer to verify robot has croseed the defense"
                    # "Drives robot forward over defense"
                    # "encoder counts"
                    n379 = call "Check Lowbar Cross.vi"() -> ("Cross"=w586:bool)  [unwired: 11 in]
                    n380 = call "Drive Straight Gyro.vi"("Distance to travel"=-1200.0) -> ()  [unwired: 10 in, 1 out]
                    n381 = Select(t=AutoStatesTypeDef."Stop" ("Defense"), s=w586, f=w587) -> (s? t:f=w589:T2)
                  }
                  frame Enabled {
                    # "Shouldn't ever be in this case in low bar auton"
                  }
                }
              }
              frame "Shoot" {
                # "Prep wheels for a set time before shooting.\nshoot. switch to stop case after 1 second"
                n382 = call "Autonomous shoot.vi"() -> ("Shot?"=w595:bool)  [unwired: 11 in]
                n383 = call "1038 Timer.vi"("Reset?"=w595, "Time Target"=2.0) -> ("Done?"=w591:bool)  [unwired: 9 in]
                n384 = Select(t=AutoStatesTypeDef."Stop" ("Defense"), s=w591, f=w593) -> (s? t:f=w592:T2)
              }
              frame "Retreat" {
                # "Maybe move wheels back?"
              }
              frame "Stop", Default {
                w598 = FALSE ("Arms.Initialize Arm Position?")
                w599 = 0.0
                # "Close Stuff"
                n385 = global read "Robot Values.vi" "Robot Values"() -> (w601:T10)
                n386 = Bundle By Name(cluster=w601, "Drive Motors.Left Motor Value"=w599, "Drive Motors.Right Motor Value"=w599, "Arms.Initialize Arm Position?"=w598, "Acquisition and Scoring.Prep Wheels"=w598, "Acquisition and Scoring.Shoot"=w598) -> (w600:T10)
                n387 = global write "Robot Values.vi" "Robot Values"(w600) -> ()
              }
              frame "Drive to defense" {
                # "Will drive straight until setpoint is reached. Need to add proper setpoint"
                n388 = call "Drive Straight Gyro.vi"("PID gains"="PID gains 4", "output range"=cluster{"output high":dbl, "output low":dbl} {"output high"=1.0, "output low"=-1.0}, "Distance to travel"=-1000.0) -> ("In Range?"=w606:bool)  [unwired: 8 in]
                n389 = Select(t=AutoStatesTypeDef."Align robot" ("Defense"), s=w606, f=w605) -> (s? t:f=w608:T2)
              }
              frame "Align robot" {
                # "Returns robot to staight position after crossing defense"
                n390 = case shown="\"First\", Default" w610 {
                  tunnel: [0.0 ("setpoint") w617 w618 w619 w620] -> w612
                  frame "First", Default {
                  }
                  frame "Second" {
                    n391 = local read "Pos 2 Align"() -> (w617:dbl)
                  }
                  frame "Third" {
                    n392 = local read "Pos 3 Align"() -> (w618:dbl)
                  }
                  frame "Fourth" {
                    n393 = local read "Pos 4 Align"() -> (w619:dbl)
                  }
                  frame "Fifth" {
                    n394 = local read "Pos 5 Align"() -> (w620:dbl)
                  }
                }
                n395 = call "Turn Angle.vi"("setpoint"=w612) -> ("In Range?"=w611:bool)  [unwired: 10 in]
                n396 = Select(t=AutoStatesTypeDef."Drive to goal" ("Defense"), s=w611, f=w615) -> (s? t:f=w614:T2)
              }
              frame "Line up to shoot" {
                n397 = call "Align to Shoot.vi"() -> ("Stop?"=w621:bool, "Aligned?"=w625:bool)  [unwired: 10 in]
                n398 = Select(t=AutoStatesTypeDef."Stop" ("Defense"), s=w621, f=w624) -> (s? t:f=w623:T2)
                n399 = Select(t=AutoStatesTypeDef."Shoot" ("Defense"), s=w625, f=w623) -> (s? t:f=w627:T2)
              }
              frame "Initialize" {
                n400 = flat-sequence {
                  tunnel: [AutoStatesTypeDef."Drive to defense" ("t")] -> w628
                  frame #0 {
                    n401 = while {
                      stop <- w632 stop-if-true
                      n402 = global read "Robot Values.vi" "Robot Values"() -> (w635:T10)
                      n403 = Unbundle By Name(w635) -> ("Arms.Left Arm Lower Limit"=w633:bool)
                      n404 = First Call?() -> (First Call?: T/F=w631:bool)
                      n405 = global read "Robot Values.vi" "Robot Values"() -> (w637:T10)
                      n406 = Bundle By Name(cluster=w637, "Sensors.Reset Gyro?"=TRUE ("Arms.Initialize Arm Position?")) -> (w636:T10)
                      n407 = call "1038 Timer.vi"("Reset?"=w631, "Time Target"=5.0) -> ("Done?"=w629:bool)  [unwired: 9 in]
                      n408 = global write "Robot Values.vi" "Robot Values"(w636) -> ()
                      n409 = Or(x=w629, y=w633) -> (x .or. y?=w632:bool)
                    }
                  }
                  frame #1 {
                    w641 = FALSE ("Arms.Initialize Arm Position?")
                    n410 = global read "Robot Values.vi" "Robot Values"() -> (w639:T10)
                    n411 = Bundle By Name(cluster=w639, "Arms.Initialize Arm Position?"=w641, "Sensors.Reset Gyro?"=w641) -> (w640:T10)
                    n412 = global write "Robot Values.vi" "Robot Values"(w640) -> ()
                  }
                }
              }
            }
          }
          frame "Drawbridge" {
          }
          frame "Sally Port" {
          }
          frame "Rock Wall" {
            n413 = disable-structure shown="Enabled" {
              disable-tunnel: w644 -> [w646 w729]
              disable-tunnel: w643 -> [w645 _]
              disable-tunnel: [_ w728] -> w642
              frame Disabled {
                n414 = case shown="\"Initialize\"" w646 {
                  selector: w646 -> [w650 w661 w669 w679 _ _ w691 w701 w710 _]
                  tunnel: [w652 w663 w670 w678 AutoStatesTypeDef."Drive to goal" ("Defense") AutoStatesTypeDef."Stop" ("Defense") w694 w700 w713 w714] -> _
                  tunnel: w645 -> [w648 w659 _ _ _ _ _ w696 _ _]
                  frame "Drive to goal" {
                    n415 = case shown="\"Fifth\"" w648 {
                      tunnel: [0.0 ("setpoint") w654 w655 w656 w657] -> w647
                      frame "First", Default {
                      }
                      frame "Second" {
                        n416 = local read "Pos 2 Drive"() -> (w654:dbl)
                      }
                      frame "Third" {
                        n417 = local read "Pos 3 Drive"() -> (w655:dbl)
                      }
                      frame "Fourth" {
                        n418 = local read "Pos 4 Drive"() -> (w656:dbl)
                      }
                      frame "Fifth" {
                        n419 = local read "Pos 5 Drive"() -> (w657:dbl)
                      }
                    }
                    n420 = call "Drive Straight Gyro.vi"("Distance to travel"=w647) -> ("In Range?"=w649:bool)  [unwired: 10 in]
                    n421 = Select(t=AutoStatesTypeDef."Turn towards goal", s=w649, f=w650) -> (s? t:f=w652:T2)
                  }
                  frame "Turn towards goal" {
                    # "Turns the robot to face toward the goal"
                    n422 = case shown="\"Fifth\"" w659 {
                      tunnel: [0.0 ("setpoint") w665 w666 w667 w668] -> w658
                      frame "First", Default {
                      }
                      frame "Second" {
                        n423 = local read "Pos 2 Turn"() -> (w665:dbl)
                      }
                      frame "Third" {
                        n424 = local read "Pos 3 Turn"() -> (w666:dbl)
                      }
                      frame "Fourth" {
                        n425 = local read "Pos 4 Turn"() -> (w667:dbl)
                      }
                      frame "Fifth" {
                        n426 = local read "Pos 5 Turn"() -> (w668:dbl)
                      }
                    }
                    n427 = call "Turn Angle.vi"("setpoint"=w658) -> ("In Range?"=w662:bool)  [unwired: 10 in]
                    n428 = Select(t=AutoStatesTypeDef."Line up to shoot" ("Defense"), s=w662, f=w661) -> (s? t:f=w663:T2)
                  }
                  frame "Cross defense" {
                    n429 = disable-structure shown="Enabled" {
                      disable-tunnel: [w675 AutoStatesTypeDef."Stop" ("Defense")] -> w670
                      disable-tunnel: w669 -> [w673 _]
                      frame Disabled {
                        # "Checks for rise and fall of accelerometer to verify robot has croseed the defense"
                        # "Drives robot forward over defense"
                        # "encoder counts"
                        n430 = call "Check Lowbar Cross.vi"() -> ("Cross"=w672:bool)  [unwired: 11 in]
                        n431 = call "Drive Straight Gyro.vi"("Distance to travel"=-1200.0) -> ()  [unwired: 10 in, 1 out]
                        n432 = Select(t=AutoStatesTypeDef."Stop" ("Defense"), s=w672, f=w673) -> (s? t:f=w675:T2)
                      }
                      frame Enabled {
                        # "Shouldn't ever be in this case in low bar auton"
                      }
                    }
                  }
                  frame "Shoot" {
                    # "Prep wheels for a set time before shooting.\nshoot. switch to stop case after 1 second"
                    n433 = call "Autonomous shoot.vi"() -> ("Shot?"=w681:bool)  [unwired: 11 in]
                    n434 = call "1038 Timer.vi"("Reset?"=w681, "Time Target"=2.0) -> ("Done?"=w677:bool)  [unwired: 9 in]
                    n435 = Select(t=AutoStatesTypeDef."Stop" ("Defense"), s=w677, f=w679) -> (s? t:f=w678:T2)
                  }
                  frame "Retreat" {
                    # "Maybe move wheels back?"
                  }
                  frame "Stop", Default {
                    w684 = FALSE ("Arms.Initialize Arm Position?")
                    w685 = 0.0
                    # "Close Stuff"
                    n436 = global read "Robot Values.vi" "Robot Values"() -> (w687:T10)
                    n437 = Bundle By Name(cluster=w687, "Drive Motors.Left Motor Value"=w685, "Drive Motors.Right Motor Value"=w685, "Arms.Initialize Arm Position?"=w684, "Acquisition and Scoring.Prep Wheels"=w684, "Acquisition and Scoring.Shoot"=w684) -> (w686:T10)
                    n438 = global write "Robot Values.vi" "Robot Values"(w686) -> ()
                  }
                  frame "Drive to defense" {
                    # "Will drive straight until setpoint is reached. Need to add proper setpoint"
                    n439 = call "Drive Straight Gyro.vi"("PID gains"="PID gains 3", "output range"=cluster{"output high":dbl, "output low":dbl} {"output high"=1.0, "output low"=-1.0}, "Distance to travel"=-1000.0) -> ("In Range?"=w692:bool)  [unwired: 8 in]
                    n440 = Select(t=AutoStatesTypeDef."Align robot" ("Defense"), s=w692, f=w691) -> (s? t:f=w694:T2)
                  }
                  frame "Align robot" {
                    # "Returns robot to staight position after crossing defense"
                    n441 = case shown="\"First\", Default" w696 {
                      tunnel: [0.0 ("setpoint") w703 w704 w705 w706] -> w698
                      frame "First", Default {
                      }
                      frame "Second" {
                        n442 = local read "Pos 2 Align"() -> (w703:dbl)
                      }
                      frame "Third" {
                        n443 = local read "Pos 3 Align"() -> (w704:dbl)
                      }
                      frame "Fourth" {
                        n444 = local read "Pos 4 Align"() -> (w705:dbl)
                      }
                      frame "Fifth" {
                        n445 = local read "Pos 5 Align"() -> (w706:dbl)
                      }
                    }
                    n446 = call "Turn Angle.vi"("setpoint"=w698) -> ("In Range?"=w697:bool)  [unwired: 10 in]
                    n447 = Select(t=AutoStatesTypeDef."Drive to goal" ("Defense"), s=w697, f=w701) -> (s? t:f=w700:T2)
                  }
                  frame "Line up to shoot" {
                    n448 = call "Align to Shoot.vi"() -> ("Stop?"=w707:bool, "Aligned?"=w711:bool)  [unwired: 10 in]
                    n449 = Select(t=AutoStatesTypeDef."Stop" ("Defense"), s=w707, f=w710) -> (s? t:f=w709:T2)
                    n450 = Select(t=AutoStatesTypeDef."Shoot" ("Defense"), s=w711, f=w709) -> (s? t:f=w713:T2)
                  }
                  frame "Initialize" {
                    n451 = flat-sequence {
                      tunnel: [AutoStatesTypeDef."Drive to defense" ("t")] -> w714
                      frame #0 {
                        n452 = while {
                          stop <- w718 stop-if-true
                          n453 = global read "Robot Values.vi" "Robot Values"() -> (w721:T10)
                          n454 = Unbundle By Name(w721) -> ("Arms.Left Arm Lower Limit"=w719:bool)
                          n455 = First Call?() -> (First Call?: T/F=w717:bool)
                          n456 = global read "Robot Values.vi" "Robot Values"() -> (w723:T10)
                          n457 = Bundle By Name(cluster=w723, "Sensors.Reset Gyro?"=TRUE ("Arms.Initialize Arm Position?")) -> (w722:T10)
                          n458 = call "1038 Timer.vi"("Reset?"=w717, "Time Target"=5.0) -> ("Done?"=w715:bool)  [unwired: 9 in]
                          n459 = global write "Robot Values.vi" "Robot Values"(w722) -> ()
                          n460 = Or(x=w715, y=w719) -> (x .or. y?=w718:bool)
                        }
                      }
                      frame #1 {
                        w727 = FALSE ("Arms.Initialize Arm Position?")
                        n461 = global read "Robot Values.vi" "Robot Values"() -> (w725:T10)
                        n462 = Bundle By Name(cluster=w725, "Arms.Initialize Arm Position?"=w727, "Sensors.Reset Gyro?"=w727) -> (w726:T10)
                        n463 = global write "Robot Values.vi" "Robot Values"(w726) -> ()
                      }
                    }
                  }
                }
              }
              frame Enabled {
                n464 = case shown="\"Stop\", Default" w729 {
                  selector: w729 -> [_ w759 _]
                  tunnel: [w730 w760 AutoStatesTypeDef."Stop" ("Defense")] -> w728
                  frame "Initialize" {
                    n465 = flat-sequence {
                      tunnel: [AutoStatesTypeDef."Drive to defense" ("t")] -> w730
                      frame #0 {
                        n466 = while {
                          stop <- w733 stop-if-true
                          n467 = disable-structure shown="Disabled" {
                            disable-tunnel: [w740 TRUE] -> w733
                            frame Disabled {
                              n468 = global read "Robot Values.vi" "Robot Values"() -> (w742:T10)
                              n469 = First Call?() -> (First Call?: T/F=w739:bool)
                              n470 = call "1038 Timer.vi"("Reset?"=w739, "Time Target"=5.0) -> ("Done?"=w737:bool)  [unwired: 9 in]
                              n471 = Unbundle By Name(w742) -> ("Arms.Left Arm Lower Limit"=w741:bool)
                              n472 = Or(x=w737, y=w741) -> (x .or. y?=w740:bool)
                            }
                            frame Enabled {
                            }
                          }
                          n473 = Wait (ms)(milliseconds to wait=u32 25) -> ()  [unwired: 1 out]
                          n474 = global read "Robot Values.vi" "Robot Values"() -> (w736:T10)
                          n475 = Bundle By Name(cluster=w736, "Arms.Initialize Arm Position?"=FALSE, "Sensors.Reset Gyro?"=TRUE ("Arms.Initialize Arm Position?")) -> (w735:T10)
                          n476 = global write "Robot Values.vi" "Robot Values"(w735) -> ()
                        }
                      }
                      frame #1 {
                        w754 = FALSE ("Arms.Initialize Arm Position?")
                        n477 = global read "Robot Global.vi" "Global Refs"() -> (w748:T11)
                        n478 = Unbundle By Name(w748) -> ("Sensor.Left Drive EncoderDevRef"=w750:T26, "Sensor.Right Drive EncoderDevRef"=w749:T26)
                        n479 = call <vilib>:"WPI_EncoderReset.vi"("EncoderDevRef"=w750) -> ("EncoderDevRef"=w747:T26)  [unwired: 9 in, 1 out]
                        n480 = call <vilib>:"WPI_EncoderReset.vi"("EncoderDevRef"=w749) -> ("EncoderDevRef"=w746:T26)  [unwired: 9 in, 1 out]
                        n481 = Wait (ms)(milliseconds to wait=u32 25) -> ()  [unwired: 1 out]
                        n482 = global read "Robot Values.vi" "Robot Values"() -> (w752:T10)
                        n483 = Bundle By Name(cluster=w752, "Arms.Initialize Arm Position?"=w754, "Sensors.Reset Gyro?"=w754) -> (w753:T10)
                        n484 = Bundle By Name(cluster=w748, "Sensor.Left Drive EncoderDevRef"=w747, "Sensor.Right Drive EncoderDevRef"=w746) -> (w745:T11)
                        n485 = global write "Robot Values.vi" "Robot Values"(w753) -> ()
                        n486 = global write "Robot Global.vi" "Global Refs"(w745) -> ()
                      }
                    }
                  }
                  frame "Drive to defense" {
                    n487 = call "Drive Straight Gyro.vi"("output range"=cluster{"output high":dbl, "output low":dbl} {"output high"=1.0, "output low"=-1.0}, "Distance to travel"=1200.0) -> ("In Range?"=w758:bool)  [unwired: 9 in]
                    n488 = Select(t=AutoStatesTypeDef."Stop", s=w758, f=w759) -> (s? t:f=w760:T2)
                  }
                  frame "Stop", Default {
                    w762 = FALSE ("Arms.Initialize Arm Position?")
                    w763 = 0.0
                    # "Close Stuff"
                    n489 = global read "Robot Values.vi" "Robot Values"() -> (w765:T10)
                    n490 = Bundle By Name(cluster=w765, "Drive Motors.Left Motor Value"=w763, "Drive Motors.Right Motor Value"=w763, "Arms.Initialize Arm Position?"=w762, "Acquisition and Scoring.Prep Wheels"=w762, "Acquisition and Scoring.Shoot"=w762) -> (w764:T10)
                    n491 = global write "Robot Values.vi" "Robot Values"(w764) -> ()
                  }
                }
              }
            }
          }
          frame "Rough Terrain" {
            n492 = disable-structure shown="Disabled" {
              disable-tunnel: w768 -> [w771 w853]
              disable-tunnel: [w770 w855] -> w767
              disable-tunnel: w766 -> [w769 w854]
              frame Disabled {
                n493 = case shown="\"Turn towards goal\"" w769 {
                  selector: w769 -> [w775 w786 w794 w804 _ _ w816 w826 w835 _]
                  tunnel: [w777 w788 w795 w803 AutoStatesTypeDef."Drive to goal" ("Defense") AutoStatesTypeDef."Stop" ("Defense") w819 w825 w838 w839] -> w770
                  tunnel: w771 -> [w773 w784 _ _ _ _ _ w821 _ _]
                  frame "Drive to goal" {
                    n494 = case shown="\"Fifth\"" w773 {
                      tunnel: [0.0 ("setpoint") "Pos 2 Drive" "Pos 3 Drive" "Pos 4 Drive" "Pos 5 Drive"] -> w772
                      frame "First", Default {
                      }
                      frame "Second" {
                      }
                      frame "Third" {
                      }
                      frame "Fourth" {
                      }
                      frame "Fifth" {
                      }
                    }
                    n495 = call "Drive Straight Gyro.vi"("Distance to travel"=w772) -> ("In Range?"=w774:bool)  [unwired: 10 in]
                    n496 = Select(t=AutoStatesTypeDef."Turn towards goal", s=w774, f=w775) -> (s? t:f=w777:T2)
                  }
                  frame "Turn towards goal" {
                    # "Turns the robot to face toward the goal"
                    n497 = case shown="\"Second\"" w784 {
                      tunnel: [0.0 ("setpoint") "Pos 2 Turn" "Pos 3 Turn" "Pos 4 Turn" "Pos 5 Turn"] -> w783
                      frame "First", Default {
                      }
                      frame "Second" {
                      }
                      frame "Third" {
                      }
                      frame "Fourth" {
                      }
                      frame "Fifth" {
                      }
                    }
                    n498 = call "Turn Angle.vi"("setpoint"=w783) -> ("In Range?"=w787:bool)  [unwired: 10 in]
                    n499 = Select(t=AutoStatesTypeDef."Line up to shoot" ("Defense"), s=w787, f=w786) -> (s? t:f=w788:T2)
                  }
                  frame "Cross defense" {
                    n500 = disable-structure shown="Enabled" {
                      disable-tunnel: [w800 AutoStatesTypeDef."Stop" ("Defense")] -> w795
                      disable-tunnel: w794 -> [w798 _]
                      frame Disabled {
                        # "Checks for rise and fall of accelerometer to verify robot has croseed the defense"
                        # "Drives robot forward over defense"
                        # "encoder counts"
                        n501 = call "Check Lowbar Cross.vi"() -> ("Cross"=w797:bool)  [unwired: 11 in]
                        n502 = call "Drive Straight Gyro.vi"("Distance to travel"=-1200.0) -> ()  [unwired: 10 in, 1 out]
                        n503 = Select(t=AutoStatesTypeDef."Stop" ("Defense"), s=w797, f=w798) -> (s? t:f=w800:T2)
                      }
                      frame Enabled {
                        # "Shouldn't ever be in this case in low bar auton"
                      }
                    }
                  }
                  frame "Shoot" {
                    # "Prep wheels for a set time before shooting.\nshoot. switch to stop case after 1 second"
                    n504 = call "Autonomous shoot.vi"() -> ("Shot?"=w806:bool)  [unwired: 11 in]
                    n505 = call "1038 Timer.vi"("Reset?"=w806, "Time Target"=2.0) -> ("Done?"=w802:bool)  [unwired: 9 in]
                    n506 = Select(t=AutoStatesTypeDef."Stop" ("Defense"), s=w802, f=w804) -> (s? t:f=w803:T2)
                  }
                  frame "Retreat" {
                    # "Maybe move wheels back?"
                  }
                  frame "Stop", Default {
                    w809 = FALSE ("Arms.Initialize Arm Position?")
                    w810 = 0.0
                    # "Close Stuff"
                    n507 = global read "Robot Values.vi" "Robot Values"() -> (w812:T10)
                    n508 = Bundle By Name(cluster=w812, "Drive Motors.Left Motor Value"=w810, "Drive Motors.Right Motor Value"=w810, "Arms.Initialize Arm Position?"=w809, "Acquisition and Scoring.Prep Wheels"=w809, "Acquisition and Scoring.Shoot"=w809) -> (w811:T10)
                    n509 = global write "Robot Values.vi" "Robot Values"(w811) -> ()
                  }
                  frame "Drive to defense" {
                    # "Will drive straight until setpoint is reached. Need to add proper setpoint"
                    n510 = call "Drive Straight Gyro.vi"("PID gains"="PID gains 2", "output range"=cluster{"output high":dbl, "output low":dbl} {"output high"=1.0, "output low"=-1.0}, "Distance to travel"=-1000.0) -> ("In Range?"=w817:bool)  [unwired: 8 in]
                    n511 = Select(t=AutoStatesTypeDef."Align robot" ("Defense"), s=w817, f=w816) -> (s? t:f=w819:T2)
                  }
                  frame "Align robot" {
                    # "Returns robot to staight position after crossing defense"
                    n512 = case shown="\"Third\"" w821 {
                      tunnel: [0.0 ("setpoint") "Pos 2 Align" "Pos 3 Align" "Pos 4 Align" "Pos 5 Align"] -> w823
                      frame "First", Default {
                      }
                      frame "Second" {
                      }
                      frame "Third" {
                      }
                      frame "Fourth" {
                      }
                      frame "Fifth" {
                      }
                    }
                    n513 = call "Turn Angle.vi"("setpoint"=w823) -> ("In Range?"=w822:bool)  [unwired: 10 in]
                    n514 = Select(t=AutoStatesTypeDef."Drive to goal" ("Defense"), s=w822, f=w826) -> (s? t:f=w825:T2)
                  }
                  frame "Line up to shoot" {
                    n515 = call "Align to Shoot.vi"() -> ("Stop?"=w832:bool, "Aligned?"=w836:bool)  [unwired: 10 in]
                    n516 = Select(t=AutoStatesTypeDef."Stop" ("Defense"), s=w832, f=w835) -> (s? t:f=w834:T2)
                    n517 = Select(t=AutoStatesTypeDef."Shoot" ("Defense"), s=w836, f=w834) -> (s? t:f=w838:T2)
                  }
                  frame "Initialize" {
                    n518 = flat-sequence {
                      tunnel: [AutoStatesTypeDef."Drive to defense" ("t")] -> w839
                      frame #0 {
                        n519 = while {
                          stop <- w843 stop-if-true
                          n520 = global read "Robot Values.vi" "Robot Values"() -> (w846:T10)
                          n521 = First Call?() -> (First Call?: T/F=w842:bool)
                          n522 = Unbundle By Name(w846) -> ("Arms.Left Arm Lower Limit"=w844:bool)
                          n523 = global read "Robot Values.vi" "Robot Values"() -> (w848:T10)
                          n524 = Bundle By Name(cluster=w848, "Sensors.Reset Gyro?"=TRUE ("Arms.Initialize Arm Position?")) -> (w847:T10)
                          n525 = call "1038 Timer.vi"("Reset?"=w842, "Time Target"=5.0) -> ("Done?"=w840:bool)  [unwired: 9 in]
                          n526 = global write "Robot Values.vi" "Robot Values"(w847) -> ()
                          n527 = Or(x=w840, y=w844) -> (x .or. y?=w843:bool)
                        }
                      }
                      frame #1 {
                        w852 = FALSE ("Arms.Initialize Arm Position?")
                        n528 = global read "Robot Values.vi" "Robot Values"() -> (w850:T10)
                        n529 = Bundle By Name(cluster=w850, "Arms.Initialize Arm Position?"=w852, "Sensors.Reset Gyro?"=w852) -> (w851:T10)
                        n530 = global write "Robot Values.vi" "Robot Values"(w851) -> ()
                      }
                    }
                  }
                }
              }
              frame Enabled {
                n531 = case shown="\"Stop\", Default" w854 {
                  selector: w854 -> [_ w890 _ w898 w905 w912]
                  tunnel: [w856 w891 AutoStatesTypeDef."Stop" ("Defense") w897 w904 w911] -> w855
                  tunnel: w853 -> [_ w884 _ _ _ _]
                  frame "Initialize" {
                    n532 = flat-sequence {
                      tunnel: [AutoStatesTypeDef."Drive to defense" ("t")] -> w856
                      frame #0 {
                        n533 = while {
                          stop <- w859 stop-if-true
                          n534 = disable-structure shown="Disabled" {
                            disable-tunnel: [w866 TRUE] -> w859
                            frame Disabled {
                              n535 = global read "Robot Values.vi" "Robot Values"() -> (w868:T10)
                              n536 = First Call?() -> (First Call?: T/F=w865:bool)
                              n537 = call "1038 Timer.vi"("Reset?"=w865, "Time Target"=5.0) -> ("Done?"=w863:bool)  [unwired: 9 in]
                              n538 = Unbundle By Name(w868) -> ("Arms.Left Arm Lower Limit"=w867:bool)
                              n539 = Or(x=w863, y=w867) -> (x .or. y?=w866:bool)
                            }
                            frame Enabled {
                            }
                          }
                          n540 = Wait (ms)(milliseconds to wait=u32 25) -> ()  [unwired: 1 out]
                          n541 = global read "Robot Values.vi" "Robot Values"() -> (w862:T10)
                          n542 = Bundle By Name(cluster=w862, "Arms.Initialize Arm Position?"=FALSE, "Sensors.Reset Gyro?"=TRUE ("Arms.Initialize Arm Position?")) -> (w861:T10)
                          n543 = global write "Robot Values.vi" "Robot Values"(w861) -> ()
                        }
                      }
                      frame #1 {
                        w880 = FALSE ("Arms.Initialize Arm Position?")
                        n544 = global read "Robot Global.vi" "Global Refs"() -> (w874:T11)
                        n545 = Unbundle By Name(w874) -> ("Sensor.Left Drive EncoderDevRef"=w876:T26, "Sensor.Right Drive EncoderDevRef"=w875:T26)
                        n546 = call <vilib>:"WPI_EncoderReset.vi"("EncoderDevRef"=w876) -> ("EncoderDevRef"=w873:T26)  [unwired: 9 in, 1 out]
                        n547 = call <vilib>:"WPI_EncoderReset.vi"("EncoderDevRef"=w875) -> ("EncoderDevRef"=w872:T26)  [unwired: 9 in, 1 out]
                        n548 = Wait (ms)(milliseconds to wait=u32 25) -> ()  [unwired: 1 out]
                        n549 = global read "Robot Values.vi" "Robot Values"() -> (w878:T10)
                        n550 = Bundle By Name(cluster=w878, "Arms.Initialize Arm Position?"=w880, "Sensors.Reset Gyro?"=w880) -> (w879:T10)
                        n551 = Bundle By Name(cluster=w874, "Sensor.Left Drive EncoderDevRef"=w873, "Sensor.Right Drive EncoderDevRef"=w872) -> (w871:T11)
                        n552 = global write "Robot Values.vi" "Robot Values"(w879) -> ()
                        n553 = global write "Robot Global.vi" "Global Refs"(w871) -> ()
                      }
                    }
                  }
                  frame "Drive to defense" {
                    n554 = Equal?(x=w884, y=T9."Third") -> (x = y?=w882:bool)
                    n555 = call "Drive Straight Gyro.vi"("output range"=cluster{"output high":dbl, "output low":dbl} {"output high"=1.0, "output low"=-1.0}, "Distance to travel"=1100.0) -> ("In Range?"=w889:bool)  [unwired: 9 in]
                    n556 = Select(t=AutoStatesTypeDef."Align robot", s=w882, f=AutoStatesTypeDef."Stop" ("t")) -> (s? t:f=w885:T2)
                    n557 = Select(t=w885, s=w889, f=w890) -> (s? t:f=w891:T2)
                  }
                  frame "Stop", Default {
                    w893 = FALSE ("Arms.Initialize Arm Position?")
                    w894 = 0.0
                    # "Close Stuff"
                    n558 = global read "Robot Values.vi" "Robot Values"() -> (w896:T10)
                    n559 = Bundle By Name(cluster=w896, "Drive Motors.Left Motor Value"=w894, "Drive Motors.Right Motor Value"=w894, "Arms.Initialize Arm Position?"=w893, "Acquisition and Scoring.Prep Wheels"=w893, "Acquisition and Scoring.Shoot"=w893) -> (w895:T10)
                    n560 = global write "Robot Values.vi" "Robot Values"(w895) -> ()
                  }
                  frame "Line up to shoot" {
                    n561 = call "Align to Shoot.vi"() -> ("Stop?"=w899:bool, "Aligned?"=w902:bool)  [unwired: 10 in]
                    n562 = Select(t=AutoStatesTypeDef."Stop" ("Defense"), s=w899, f=w898) -> (s? t:f=w901:T2)
                    n563 = Select(t=AutoStatesTypeDef."Shoot" ("Defense"), s=w902, f=w901) -> (s? t:f=w897:T2)
                  }
                  frame "Align robot" {
                    n564 = disable-structure shown="Enabled" {
                      disable-tunnel: [w909 180.0 ("Pos 3 Align")] -> w906
                      frame Disabled {
                        n565 = local read item#-1() -> (w909)
                      }
                      frame Enabled {
                      }
                    }
                    n566 = call "Turn Angle.vi"("setpoint"=w906) -> ("In Range?"=w907:bool)  [unwired: 10 in]
                    n567 = Select(t=AutoStatesTypeDef."Line up to shoot" ("Defense"), s=w907, f=w905) -> (s? t:f=w904:T2)
                  }
                  frame "Shoot" {
                    # "Prep wheels for a set time before shooting.\nshoot. switch to stop case after 1 second"
                    n568 = call "Autonomous shoot.vi"() -> ("Shot?"=w913:bool)  [unwired: 11 in]
                    n569 = Select(t=AutoStatesTypeDef."Stop" ("Defense"), s=w913, f=w912) -> (s? t:f=w911:T2)
                  }
                }
              }
            }
          }
          frame "Low Bar" {
            n570 = case shown="\"Drive to goal\"" w915 {
              selector: w915 -> [w919 w946 w949 w959 _ _ _ w993 w1008 _ _ w1022]
              tunnel: [w920 w948 w950 w958 AutoStatesTypeDef."Drive to goal" ("Defense") AutoStatesTypeDef."Stop" ("Defense") w968 w992 w1011 w1012 _ w1021] -> w916
              frame "Drive to goal" {
                n571 = flat-sequence {
                  tunnel: [w934] -> w917
                  tunnel: [w943] -> w918
                  tunnel: w917 -> [w943]
                  frame #0 {
                    n572 = global read "Robot Global.vi" "Global Refs"() -> (w931:T11)
                    n573 = Unbundle By Name(w931) -> ("Sensor.Left Drive EncoderDevRef"=w933:T26, "Sensor.Right Drive EncoderDevRef"=w932:T26)
                    n574 = call <vilib>:"WPI_EncoderReset.vi"("EncoderDevRef"=w933) -> ("EncoderDevRef"=w930:T26)  [unwired: 9 in, 1 out]
                    n575 = call <vilib>:"WPI_EncoderReset.vi"("EncoderDevRef"=w932) -> ("EncoderDevRef"=w929:T26)  [unwired: 9 in, 1 out]
                    n576 = Wait (ms)(milliseconds to wait=u32 25) -> ()  [unwired: 1 out]
                    n577 = Bundle By Name(cluster=w931, "Sensor.Left Drive EncoderDevRef"=w930, "Sensor.Right Drive EncoderDevRef"=w929) -> (w928:T11)
                    n578 = global write "Robot Global.vi" "Global Refs"(w928) -> ()
                  }
                  frame #1 {
                    n579 = while {
                      tunnel: [w935] -> w934
                      stop <- w937 stop-if-true
                      n580 = call "Drive Straight Gyro.vi"("Distance to travel"=-101.0) -> ("In Range?"=w937:bool)  [unwired: 10 in]
                      n581 = Select(t=AutoStatesTypeDef."Line up to shoot" ("Defense"), s=w937, f=AutoStatesTypeDef."Drive to goal") -> (s? t:f=w935:T2)
                      n582 = call "Auton Reaquire.vi"() -> ()  [unwired: 12 in]
                    }
                  }
                  frame #2 {
                    w940 = 0.0
                    n583 = global read "Robot Values.vi" "Robot Values"() -> (w941:T10)
                    n584 = Bundle By Name(cluster=w941, "Drive Motors.Left Motor Value"=w940, "Drive Motors.Right Motor Value"=w940) -> (w942:T10)
                    n585 = global write "Robot Values.vi" "Robot Values"(w942) -> ()
                  }
                }
                n586 = disable-structure shown="Enabled" {
                  disable-tunnel: [w925 w926] -> w920
                  disable-tunnel: w919 -> [w923 _]
                  disable-tunnel: w918 -> [_ w926]
                  frame Disabled {
                    n587 = call "Drive Straight Gyro.vi"("Distance to travel"=-150.0) -> ("In Range?"=w922:bool)  [unwired: 10 in]
                    n588 = Select(t=AutoStatesTypeDef."Line up to shoot", s=w922, f=w923) -> (s? t:f=w925:T2)
                  }
                  frame Enabled {
                  }
                }
              }
              frame "Turn towards goal" {
                # "Turns the robot to face toward the goal"
                n589 = call "Turn Angle.vi"("setpoint"=45.0) -> ("In Range?"=w947:bool)  [unwired: 10 in]
                n590 = Select(t=AutoStatesTypeDef."Line up to shoot" ("Defense"), s=w947, f=w946) -> (s? t:f=w948:T2)
              }
              frame "Cross defense" {
                n591 = disable-structure shown="Disabled" {
                  disable-tunnel: [w955 AutoStatesTypeDef."Stop" ("Defense")] -> w950
                  disable-tunnel: w949 -> [w953 _]
                  frame Disabled {
                    # "Checks for rise and fall of accelerometer to verify robot has croseed the defense"
                    # "Drives robot forward over defense"
                    # "encoder counts"
                    n592 = call "Check Lowbar Cross.vi"() -> ("Cross"=w952:bool)  [unwired: 11 in]
                    n593 = call "Drive Straight Gyro.vi"("Distance to travel"=-1400.0) -> ()  [unwired: 10 in, 1 out]
                    n594 = Select(t=AutoStatesTypeDef."Align robot" ("Defense"), s=w952, f=w953) -> (s? t:f=w955:T2)
                  }
                  frame Enabled {
                    # "Shouldn't ever be in this case in low bar auton"
                  }
                }
              }
              frame "Shoot" {
                # "Prep wheels for a set time before shooting.\nshoot. switch to stop case after 1 second"
                n595 = call "Autonomous shoot.vi"() -> ("Shot?"=w957:bool)  [unwired: 11 in]
                n596 = Select(t=AutoStatesTypeDef."Stop" ("Defense"), s=w957, f=w959) -> (s? t:f=w958:T2)
              }
              frame "Retreat" {
                # "Maybe move wheels back?"
              }
              frame "Stop", Default {
                w962 = FALSE ("Arms.Initialize Arm Position?")
                w963 = 0.0
                # "Close Stuff"
                n597 = global read "Robot Values.vi" "Robot Values"() -> (w965:T10)
                n598 = Bundle By Name(cluster=w965, "Drive Motors.Left Motor Value"=w963, "Drive Motors.Right Motor Value"=w963, "Arms.Initialize Arm Position?"=w962, "Acquisition and Scoring.Shoot"=w962, "Acquisition and Scoring.Prep Wheels"=w962) -> (w964:T10)
                n599 = global write "Robot Values.vi" "Robot Values"(w964) -> ()
              }
              frame "Drive to defense" {
                # "Will drive straight until setpoint is reached. Need to add proper setpoint"
                n600 = flat-sequence {
                  tunnel: [w976] -> w967
                  tunnel: [w989] -> w968
                  tunnel: w967 -> [w989]
                  frame #0 {
                    n601 = global read "Robot Global.vi" "Global Refs"() -> (w973:T11)
                    n602 = Unbundle By Name(w973) -> ("Sensor.Left Drive EncoderDevRef"=w975:T26, "Sensor.Right Drive EncoderDevRef"=w974:T26)
                    n603 = call <vilib>:"WPI_EncoderReset.vi"("EncoderDevRef"=w975) -> ("EncoderDevRef"=w972:T26)  [unwired: 9 in, 1 out]
                    n604 = call <vilib>:"WPI_EncoderReset.vi"("EncoderDevRef"=w974) -> ("EncoderDevRef"=w971:T26)  [unwired: 9 in, 1 out]
                    n605 = Wait (ms)(milliseconds to wait=u32 25) -> ()  [unwired: 1 out]
                    n606 = Bundle By Name(cluster=w973, "Sensor.Left Drive EncoderDevRef"=w972, "Sensor.Right Drive EncoderDevRef"=w971) -> (w970:T11)
                    n607 = global write "Robot Global.vi" "Global Refs"(w970) -> ()
                  }
                  frame #1 {
                    n608 = while {
                      tunnel: [w979] -> w976
                      stop <- w981 stop-if-true
                      n609 = Wait (ms)(milliseconds to wait=u32 1) -> ()  [unwired: 1 out]
                      n610 = call "Drive Straight Gyro.vi"("output range"=cluster{"output high":dbl, "output low":dbl} {"output high"=0.6, "output low"=-0.6}, "Distance to travel"=-1450.0) -> ("In Range?"=w981:bool)  [unwired: 9 in]
                      n611 = Select(t=AutoStatesTypeDef."Raise Arms" ("Defense"), s=w981, f=AutoStatesTypeDef."Drive to defense") -> (s? t:f=w979:T2)
                      n612 = call "Auton Reaquire.vi"() -> ()  [unwired: 12 in]
                    }
                  }
                  frame #2 {
                    w985 = 0.0
                    n613 = global read "Robot Values.vi" "Robot Values"() -> (w986:T10)
                    n614 = Bundle By Name(cluster=w986, "Drive Motors.Left Motor Value"=w985, "Drive Motors.Right Motor Value"=w985, "Arms.Initialize Arm Position?"=FALSE) -> (w987:T10)
                    n615 = Wait (ms)(milliseconds to wait=u32 500) -> ()  [unwired: 1 out]
                    n616 = global write "Robot Values.vi" "Robot Values"(w987) -> ()
                  }
                }
              }
              frame "Align robot" {
                # "Returns robot to staight position after crossing defense"
                n617 = flat-sequence {
                  tunnel: [w1000] -> w990
                  frame #0 {
                    n618 = while {
                      stop <- w994 stop-if-true
                      n619 = call "Turn Angle.vi"("setpoint"=50.0) -> ("In Range?"=w994:bool)  [unwired: 10 in]
                    }
                  }
                  frame #1 {
                    w996 = 0.0
                    n620 = global read "Robot Values.vi" "Robot Values"() -> (w997:T10)
                    n621 = Bundle By Name(cluster=w997, "Drive Motors.Left Motor Value"=w996, "Drive Motors.Right Motor Value"=w996) -> (w998:T10)
                    n622 = Wait (ms)(milliseconds to wait=u32 500) -> ()  [unwired: 1 out]
                    n623 = global write "Robot Values.vi" "Robot Values"(w998) -> ()
                  }
                  frame #2 {
                    n624 = global read "Robot Values.vi" "Robot Values"() -> (w1004:T10)
                    n625 = Unbundle By Name(w1004) -> ("Sensors.Gyro Angle"=w1003:dbl)
                    n626 = In Range and Coerce(upper limit=50.5, x=w1003, lower limit=49.5 ("x")) -> (In Range?=w1000:bool)  [unwired: 1 out]
                  }
                }
                n627 = Select(t=AutoStatesTypeDef."Drive to goal" ("Defense"), s=w990, f=w993) -> (s? t:f=w992:T2)
              }
              frame "Line up to shoot" {
                n628 = call "Align to Shoot.vi"() -> ("Stop?"=w1005:bool, "Aligned?"=w1009:bool)  [unwired: 10 in]
                n629 = Select(t=AutoStatesTypeDef."Stop" ("Defense"), s=w1005, f=w1008) -> (s? t:f=w1007:T2)
                n630 = Select(t=AutoStatesTypeDef."Shoot" ("Defense"), s=w1009, f=w1007) -> (s? t:f=w1011:T2)
              }
              frame "Initialize" {
                n631 = flat-sequence {
                  tunnel: [AutoStatesTypeDef."Drive to defense" ("t")] -> w1012
                  frame #0 {
                    w1014 = TRUE ("Arms.Initialize Arm Position?")
                    n632 = global read "Robot Values.vi" "Robot Values"() -> (w1016:T10)
                    n633 = Bundle By Name(cluster=w1016, "Arms.Initialize Arm Position?"=w1014, "Sensors.Reset Gyro?"=w1014) -> (w1015:T10)
                    n634 = Wait (ms)(milliseconds to wait=u32 20) -> ()  [unwired: 1 out]
                    n635 = global write "Robot Values.vi" "Robot Values"(w1015) -> ()
                  }
                  frame #1 {
                    w1017 = FALSE ("Arms.Initialize Arm Position?")
                    n636 = global read "Robot Values.vi" "Robot Values"() -> (w1019:T10)
                    n637 = Bundle By Name(cluster=w1019, "Sensors.Reset Gyro?"=w1017, "Acquisition and Scoring.Prep Wheels"=w1017) -> (w1020:T10)
                    n638 = global write "Robot Values.vi" "Robot Values"(w1020) -> ()
                  }
                }
              }
              frame "Lower Arms" {
              }
              frame "Raise Arms" {
                n639 = First Call?() -> (First Call?: T/F=w1030:bool)
                n640 = call "1038 Timer.vi"("Reset?"=w1030, "Time Target"=1.0) -> ("Done?"=w1024:bool)  [unwired: 9 in]
                n641 = Select(t=0.0, s=w1024, f=-1.0) -> (s? t:f=w1031:dbl)
                n642 = global read "Robot Values.vi" "Robot Values"() -> (w1025:T10)
                n643 = Bundle By Name(cluster=w1025, "Arms.Desired Arm Position"=w1031) -> (w1026:T10)
                n644 = global write "Robot Values.vi" "Robot Values"(w1026) -> ()
                n645 = Select(t=AutoStatesTypeDef."Align robot" ("Defense"), s=w1024, f=w1022) -> (s? t:f=w1021:T2)
              }
            }
          }
          frame "None", Default {
          }
          frame "Reach" {
            n646 = case shown="\"Stop\", Default" w1033 {
              selector: w1033 -> [_ w1062 _]
              tunnel: [w1034 w1063 AutoStatesTypeDef."Stop" ("Defense")] -> w1032
              frame "Initialize" {
                n647 = flat-sequence {
                  tunnel: [AutoStatesTypeDef."Drive to defense" ("t")] -> w1034
                  frame #0 {
                    n648 = while {
                      stop <- w1037 stop-if-true
                      n649 = disable-structure shown="Disabled" {
                        disable-tunnel: [w1044 TRUE] -> w1037
                        frame Disabled {
                          n650 = global read "Robot Values.vi" "Robot Values"() -> (w1046:T10)
                          n651 = First Call?() -> (First Call?: T/F=w1043:bool)
                          n652 = call "1038 Timer.vi"("Reset?"=w1043, "Time Target"=5.0) -> ("Done?"=w1041:bool)  [unwired: 9 in]
                          n653 = Unbundle By Name(w1046) -> ("Arms.Left Arm Lower Limit"=w1045:bool)
                          n654 = Or(x=w1041, y=w1045) -> (x .or. y?=w1044:bool)
                        }
                        frame Enabled {
                        }
                      }
                      n655 = Wait (ms)(milliseconds to wait=u32 25) -> ()  [unwired: 1 out]
                      n656 = global read "Robot Values.vi" "Robot Values"() -> (w1040:T10)
                      n657 = Bundle By Name(cluster=w1040, "Arms.Initialize Arm Position?"=FALSE, "Sensors.Reset Gyro?"=TRUE ("Arms.Initialize Arm Position?")) -> (w1039:T10)
                      n658 = global write "Robot Values.vi" "Robot Values"(w1039) -> ()
                    }
                  }
                  frame #1 {
                    w1058 = FALSE ("Arms.Initialize Arm Position?")
                    n659 = global read "Robot Global.vi" "Global Refs"() -> (w1052:T11)
                    n660 = Unbundle By Name(w1052) -> ("Sensor.Left Drive EncoderDevRef"=w1054:T26, "Sensor.Right Drive EncoderDevRef"=w1053:T26)
                    n661 = call <vilib>:"WPI_EncoderReset.vi"("EncoderDevRef"=w1054) -> ("EncoderDevRef"=w1051:T26)  [unwired: 9 in, 1 out]
                    n662 = call <vilib>:"WPI_EncoderReset.vi"("EncoderDevRef"=w1053) -> ("EncoderDevRef"=w1050:T26)  [unwired: 9 in, 1 out]
                    n663 = Wait (ms)(milliseconds to wait=u32 25) -> ()  [unwired: 1 out]
                    n664 = global read "Robot Values.vi" "Robot Values"() -> (w1056:T10)
                    n665 = Bundle By Name(cluster=w1056, "Arms.Initialize Arm Position?"=w1058, "Sensors.Reset Gyro?"=w1058) -> (w1057:T10)
                    n666 = Bundle By Name(cluster=w1052, "Sensor.Left Drive EncoderDevRef"=w1051, "Sensor.Right Drive EncoderDevRef"=w1050) -> (w1049:T11)
                    n667 = global write "Robot Values.vi" "Robot Values"(w1057) -> ()
                    n668 = global write "Robot Global.vi" "Global Refs"(w1049) -> ()
                  }
                }
              }
              frame "Drive to defense" {
                n669 = call "Drive Straight Gyro.vi"("Distance to travel"=235.0) -> ("In Range?"=w1061:bool)  [unwired: 10 in]
                n670 = Select(t=AutoStatesTypeDef."Stop", s=w1061, f=w1062) -> (s? t:f=w1063:T2)
              }
              frame "Stop", Default {
                w1065 = FALSE ("Arms.Initialize Arm Position?")
                w1066 = 0.0
                # "Close Stuff"
                n671 = global read "Robot Values.vi" "Robot Values"() -> (w1068:T10)
                n672 = Bundle By Name(cluster=w1068, "Drive Motors.Left Motor Value"=w1066, "Drive Motors.Right Motor Value"=w1066, "Arms.Initialize Arm Position?"=w1065, "Acquisition and Scoring.Prep Wheels"=w1065, "Acquisition and Scoring.Shoot"=w1065) -> (w1067:T10)
                n673 = global write "Robot Values.vi" "Robot Values"(w1067) -> ()
              }
            }
          }
          frame "Spy Bot" {
          }
        }
        n674 = Wait (ms)(milliseconds to wait=u32 1) -> ()  [unwired: 1 out]
      }
    }
    frame Disabled {
    }
  }
  n675 = disable-structure shown="Enabled" {
    disable-tunnel: w3 -> [w1069 _]
    frame Disabled {
      # "Use time and/or sensors to control how the robot drives."
      n676 = case shown="\"Alternative 1\"" w1069 {
        frame Default {
          # "You can put your main auto here, or you can right-click on the case and make any\nother frame be the default case."
          # "This is the frame that will execute if no selection is made, or if it is not recognized"
        }
        frame "Alternative 1" {
          # "This sample code describes robot movements in an array. You can extend it to control other motors\non your robot. You can also use file I/O to move the data to a text file."
          n677 = call <vilib>:"WPI_RobotDriveRefNum Registry Get.vi"("refnum name"="Left and Right Motors") -> ("RobotDriveDevRef"=w1071:T12)  [unwired: 1 in, 9 out]
          n678 = for {
            shift-right: [w1079] -> _
            shift-left: w1071 -> [w1080]
            tunnel: "Array of robot movements" -> [w1075] mode=indexing
            n679 = Unbundle By Name(w1075) -> ("X Joystick Value"=w1078:dbl, "Y Joystick Value"=w1077:dbl, "Delay (sec)"=w1076:dbl)  [unwired: 1 out]
            n680 = call-poly <vilib>:"WPI_RobotDriveArcadeDrive.vi"("Y axis value"=w1077, "X axis value"=w1078, "RobotDriveDevRef"=w1080) -> ("Motor Values"=w1073:dbl[], "RobotDriveDevRef"=w1081:T12)  [unwired: 1 in, 6 out]
            n681 = call-poly <vilib>:"NT Write Value.vi"("Numeric Array"=w1073, "Name"="RobotDrive Motors") -> ()  [unwired: 9 in, 1 out]
            n682 = call <vilib>:"WPI_RobotDriveDelayAndUpdateSafety.vi"("Delay (s)"=w1076, "RobotDriveDevRef"=w1081) -> ("RobotDriveDevRef 2"=w1079:T12)  [unwired: 8 in, 1 out]
            "Current Movement, for debugging" <- w1075
          }
        }
        frame "Alternative 2" {
          w1083 = "RobotDrive Motors" ("Name")
          # "This is some simple sample code to drive your robot curving one direction and then the other."
          # "stand still"
          # "other way for 0.5 second"
          # "turn for 1 second"
          n683 = call <vilib>:"WPI_RobotDriveRefNum Registry Get.vi"("refnum name"="Left and Right Motors") -> ("RobotDriveDevRef"=w1099:T12)  [unwired: 1 in, 9 out]
          n684 = call-poly <vilib>:"WPI_RobotDriveArcadeDrive.vi"("Y axis value"=0.5 ("X axis value"), "X axis value"=-0.25, "RobotDriveDevRef"=w1099) -> ("Motor Values"=w1082:dbl[], "RobotDriveDevRef"=w1092:T12)  [unwired: 1 in, 6 out]
          n685 = call-poly <vilib>:"NT Write Value.vi"("Numeric Array"=w1082, "Name"=w1083) -> ()  [unwired: 9 in, 1 out]
          n686 = call <vilib>:"WPI_RobotDriveDelayAndUpdateSafety.vi"("Delay (s)"=1.0, "RobotDriveDevRef"=w1092) -> ("RobotDriveDevRef 2"=w1093:T12)  [unwired: 8 in, 1 out]
          n687 = call-poly <vilib>:"WPI_RobotDriveArcadeDrive.vi"("Y axis value"=-0.25 ("X axis value"), "X axis value"=0.5, "RobotDriveDevRef"=w1093) -> ("Motor Values"=w1084:dbl[], "RobotDriveDevRef"=w1094:T12)  [unwired: 1 in, 6 out]
          n688 = call-poly <vilib>:"NT Write Value.vi"("Numeric Array"=w1084, "Name"=w1083) -> ()  [unwired: 9 in, 1 out]
          n689 = call <vilib>:"WPI_RobotDriveDelayAndUpdateSafety.vi"("Delay (s)"=0.5, "RobotDriveDevRef"=w1094) -> ("RobotDriveDevRef 2"=w1095:T12)  [unwired: 8 in, 1 out]
          n690 = call-poly <vilib>:"WPI_RobotDriveArcadeDrive.vi"("Y axis value"=0.0 ("X axis value"), "X axis value"=0.0, "RobotDriveDevRef"=w1095) -> ("Motor Values"=w1085:dbl[])  [unwired: 1 in, 7 out]
          n691 = call-poly <vilib>:"NT Write Value.vi"("Numeric Array"=w1085, "Name"=w1083) -> ()  [unwired: 9 in, 1 out]
        }
        frame "Your Turn" {
        }
      }
    }
    frame Enabled {
      n692 = disable-structure shown="Disabled" {
        frame Disabled {
          n693 = while {
            stop <- _ stop-if-true
            (unwired) 90.0 ("setpoint")
            (unwired) T1 {"proportional gain (Kc)"=0.06, "integral time (Ti, min)"=0.0, "derivative time (Td, min)"=0.0} ("PID gains")
            (unwired) cluster{"output high":dbl, "output low":dbl} {"output high"=0.6, "output low"=-0.6} ("output range")
            n694 = global read "Robot Values.vi" "Robot Values"() -> (w1102:T10)
            n695 = Unbundle By Name(w1102) -> ("Sensors.Gyro Angle"=w1104:dbl)
            n696 = Quotient & Remainder(x=w1104, y=360.0) -> (x-y*floor(x/y)=w1100:dbl)  [unwired: 1 out]
            n697 = call "Turn Angle.vi"("setpoint"=w1100) -> ()  [unwired: 10 in, 1 out]
            n698 = Bundle By Name(cluster=w1102) -> (w1101:T10)  [unwired: 2 in]
            n699 = global write "Robot Values.vi" "Robot Values"(w1101) -> ()
          }
        }
        frame Enabled {
        }
      }
    }
  }
